vi "WF phase diversity_MATLAB_Correction_loop_AndorSDK_imq.vi"() -> ()   [LabVIEW 2018]
uses:
  <userlib>/WaveKit.lib/Controls/Wavefront Corrector states - ONE.ctl
  <userlib>/WaveKit.lib/Classes/WavefrontCorrector/WavefrontCorrector.lvclass
  <userlib>/WaveKit.lib/Classes/WavefrontCorrectorSet/WavefrontCorrectorSet.lvclass
  <vilib>/Analysis/1siggen.llb/Ramp Pattern by Samples.vi
  <vilib>/Utility/file.llb/Read From Spreadsheet File (DBL).vi
  <vilib>/Analysis/1siggen.llb/Ramp Pattern by Delta.vi
  <vilib>/Analysis/NI_AALBase.lvlib
panel:
  in  "Tab Control":T1(tab)
  in  "Offset command file":path=path "D:/SystemAlignment/system_aberration_20200627.dat"
  in  "Initial haso file":path=path "D:/SystemAlignment/system_aberration_residual_20200711.has"
  out "# of Phase":i32
  in  "DM configuration file":path=path "C:/Program Files (x86)/Imagine Optic/Configuration Files/WaveFrontCorrector_mirao52-e_0326.dat"
  out "DM Initial State":T2[](array[typedef])
  out "DM ActuatorsNumber":i32
  out "Error out":errorcluster
  in  "EMCCD trigger port":tag="Dev1/port0/line0"
  in  "COMMAND matrix path":path=path "D:/SystemAlignment/CM_20200711_0p5x6.aomc"
  out "Detector Y Pixels":i32
  out "Detector X Pixels":i32
  out "Return from Initialize":u32
  out "Return from SetTemperature":u32
  out "Calculated Exposure Value":sgl format="%.2f"
  out "Return from CheckTimings":u32
  in  "488 shutter":refnum<k7>(container)
  in  "?":bool
  in  "Initial Zer coeff":dbl[](array[numeric])=[0.2, 0.2]
  in  "Initial Zer index":dbl[](array[numeric])=[4.0, 5.0]
  out "Initial Zer coeff\nRandomly generated":dbl[](array[numeric])
  out "Initial Zer index (starting from 4)\nrandomly generated":dbl[](array[numeric])
  in  "aberration tolerance":dbl=0.1 format="%#_13g"
  in  "aberration threshold":dbl=0.25 format="%#_13g"
  in  "Initial Zern Coefficients":enum16{"input manually ", "randomly generated"}(ring)
  in  "max random order":i64=9
  in  "NOT YET: Data Acquisition Iteration #":i32=1
  in  "Index 5":i32[](array[numeric])=[3, 4, 5, 6, 7, 8]
  in  "Coef 4":sgl[](array[numeric])=[0.2, 0.0, 0.0, 0.0, 0.0, 0.0]
  in  "Index 4":i32[](array[numeric])=[3, 4, 5, 6, 7, 8]
  in  "Coef 3":sgl[](array[numeric])=[-0.2, -0.5, 0.0, 0.0, 0.0, 0.0]
  in  "Index 3":i32[](array[numeric])=[3, 4, 5, 6, 7, 8]
  in  "Coef 2":sgl[](array[numeric])=[0.2, 0.5, 0.0, 0.0, 0.0, 0.0]
  in  "Index 2":i32[](array[numeric])=[3, 4, 5, 6, 7, 8]
  in  "Zern coef in 5":sgl[](array[numeric])=[-0.2, 0.5, 0.0, 0.0, 0.0, 0.0]
  in  "base name":string="beads_test"
  in  "Imgs/phase":dbl=1.0
  in  "camera exposure time (s)":string="0.02"
  in  "# of Phase":i32=5
  in  "number of phase div image":dbl(ring)=2.0 items=["adding by step of 1 image"=1.0, "jump to 3 images"=0.9, "jump to 4 images"=2.0, "jump to 5 images"=2.9]
  in  "Metrics Type":T3(ring)=enum."norm DCT  - spectral domain 3: 0~r0"
  in  "Keep Reconstructed Defocus component?":bool
  in  "Run MATLAB or correction?":bool=TRUE
  in  "Number for average":u32=1
  in  "Zernike Order":u32=20
  in  "Iteration Number":u32=10
  in  "Gamma Value":dbl=1e-06
  in  "Crop Size of image":u32=512
  in  "Background Value":u32=290
  in  "Show Input":bool
  in  "Show Recon":bool=TRUE
  in  "Use GPU":bool=TRUE
  out "Cooling":i32
  in  "Trigger":u32(ring)=1 items=["Internal", "External"]
  in  "Cooler set to Temperature":i32=-60
  in  "Initialize EMCCD?":bool=TRUE
  in  "Turn off EMCCD when finished?":bool
  in  "Main Path":path=path "D:/Data"
  in  "Subfolder":string="Sample1"
  in  "Folder Name":string="Test"
  out "groundtruth image quality value":dbl
  out "aberrated image quality value":dbl
  out "Corrected Image Quality Value":dbl[](array[numeric])
  # "priority:\n1, flip, done by Min on 20200731? \n2, organize\n3, new matlab PD code\n4. isolate shutdown\n5. add \"galvo to andor\"\n6. setting log\n\n\n\n2 PhasDiv first\nif not, take 3 more or start over 5\n\n??: random iteration work??\n\nadd preview"
  # "If Pics/phase is 2:\npicture order:\n\noffset+aberr *2\nphase diversity *8\n\nground truth *1\noffset+aberr *1\ncorrected *2 but the last one cannot be seen in imagej"
  # "Andor Status"
  # "Random Input"
  # "Manual Input"
  # "Manual input sequence"
  # "Andor Camera Settings"
  # "Andor EMCCD Settings"
  # "MATLAB Settings"
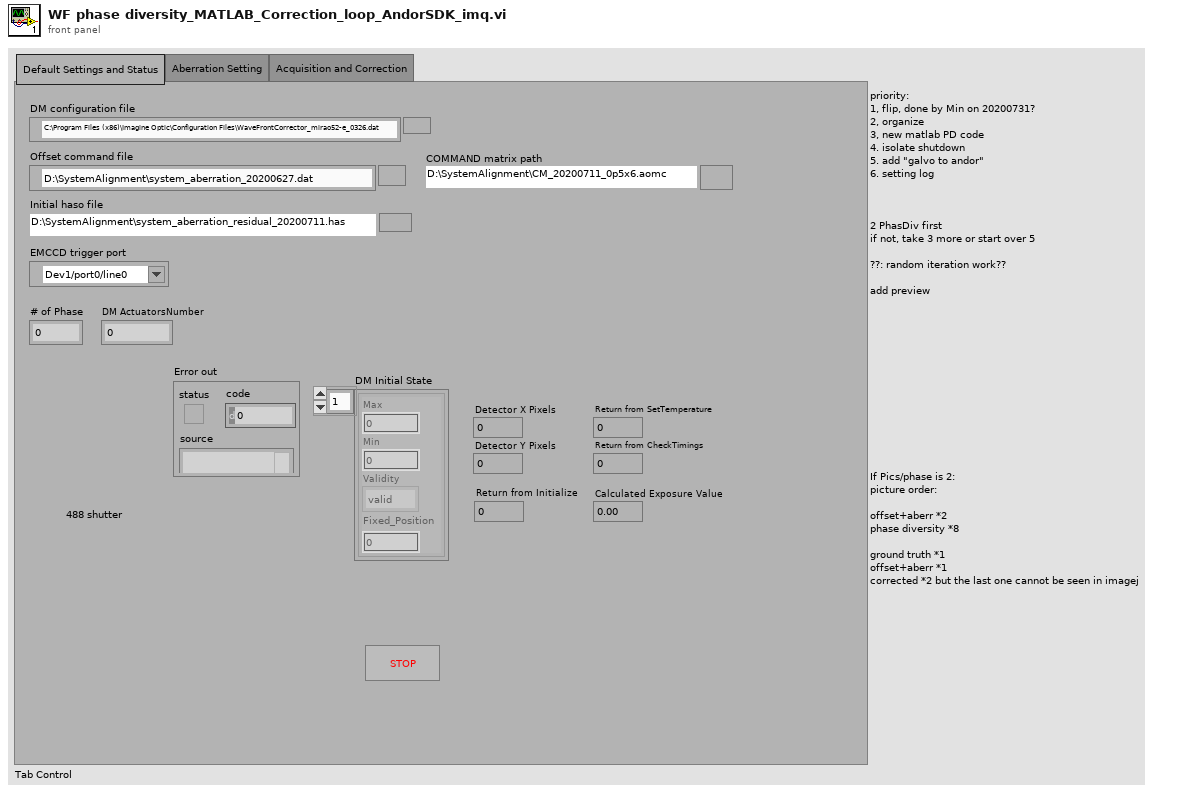
[diagram p1: front panel]
types:
  T1 = enum32{"Default Settings and Status", "Aberration Setting", "Acquisition and Correction"}
  T2 = typedef "Wavefront Corrector states - ONE.ctl" = cluster{"Max":sgl, "Min":sgl, "Validity":enum16{"valid", "fixed", "invalid"}, "Fixed_Position":sgl}
  T3 = enum16{" ", "max intensity", "mean intensity", "RMS contrast", "sharpness - image domain", "sharpness - spectral domain 1: 0~r0", "sharpness - spectral domain 2: 0.1*r0~0.5*r0", "norm DCT  - spectral domain 3: 0~r0"}
  T4 = typedef "Error Code Enum typedef.ctl" = enum32{"N/A (0)", "DRV_ERROR_CODES", "DRV_SUCCESS", "DRV_VXDNOTINSTALLED", "DRV_ERROR_SCAN", "DRV_ERROR_CHECK_SUM", "DRV_ERROR_FILELOAD", "DRV_UNKNOWN_FUNC", "DRV_ERROR_VXD_INIT", "DRV_ERROR_ADDRESS", "DRV_ERROR_PAGELOCK", "DRV_ERROR_PAGEUNLOCK", "DRV_ERROR_BOARDTEST", "DRV_ERROR_ACK", "DRV_ERROR_UP_FIFO", "DRV_ERROR_PATTERN", "N/A (16)", "DRV_ACQUISITION_ERRORS", "DRV_ACQ_BUFFER", "DRV_ACQ_DOWNFIFO_FULL", "DRV_PROC_UNKONWN_INSTRUCTION", "DRV_ILLEGAL_OP_CODE", "DRV_KINETIC_TIME_NOT_MET", "DRV_ACCUM_TIME_NOT_MET", "DRV_NO_NEW_DATA", "N/A (25)", "DRV_SPOOLERROR", "N/A (27)", "N/A (28)", "N/A (29)", "N/A (30)", "N/A (31)", "N/A (32)", "DRV_TEMPERATURE_CODES", "DRV_TEMPERATURE_OFF", "DRV_TEMPERATURE_NOT_STABILIZED", "DRV_TEMPERATURE_STABILIZED", "DRV_TEMPERATURE_NOT_REACHED", "DRV_TEMPERATURE_OUT_RANGE", "DRV_TEMPERATURE_NOT_SUPPORTED", "DRV_TEMPERATURE_DRIFT", "N/A (41)", "N/A (42)", "N/A (43)", "N/A (44)", "N/A (45)", "N/A (46)", "N/A (47)", "N/A (48)", "DRV_GENERAL_ERRORS", "DRV_INVALID_AUX", "DRV_COF_NOTLOADED", "DRV_FPGAPROG", "DRV_FLEXERROR", "DRV_GPIBERROR", "N/A (55)", "N/A (56)", "N/A (57)", "N/A (58)", "N/A (59)", "N/A (60)", "N/A (61)", "N/A (62)", "N/A (63)", "DRV_DATATYPE", "DRV_DRIVER_ERRORS", "DRV_P1INVALID", "DRV_P2INVALID", "DRV_P3INVALID", "DRV_P4INVALID", "DRV_INIERROR", "DRV_COFERROR", "DRV_ACQUIRING", "DRV_IDLE", "DRV_TEMPCYCLE", "DRV_NOT_INITIALIZED", "DRV_P5INVALID", "DRV_P6INVALID", "DRV_INVALID_MODE", "DRV_INVALID_FILTER", "DRV_I2CERRORS", "DRV_I2CDEVNOTFOUND", "DRV_I2CTIMEOUT", "DRV_P7INVALID", "N/A (84)", "N/A (85)", "N/A (86)", "N/A (87)", "N/A (88)", "N/A (89)", "DRV_IOCERROR", "DRV_VRMVERSIONERROR"}
  T5 = typedef "NI_Matrix.lvlib/RealMatrix.ctl" = dbl[][]
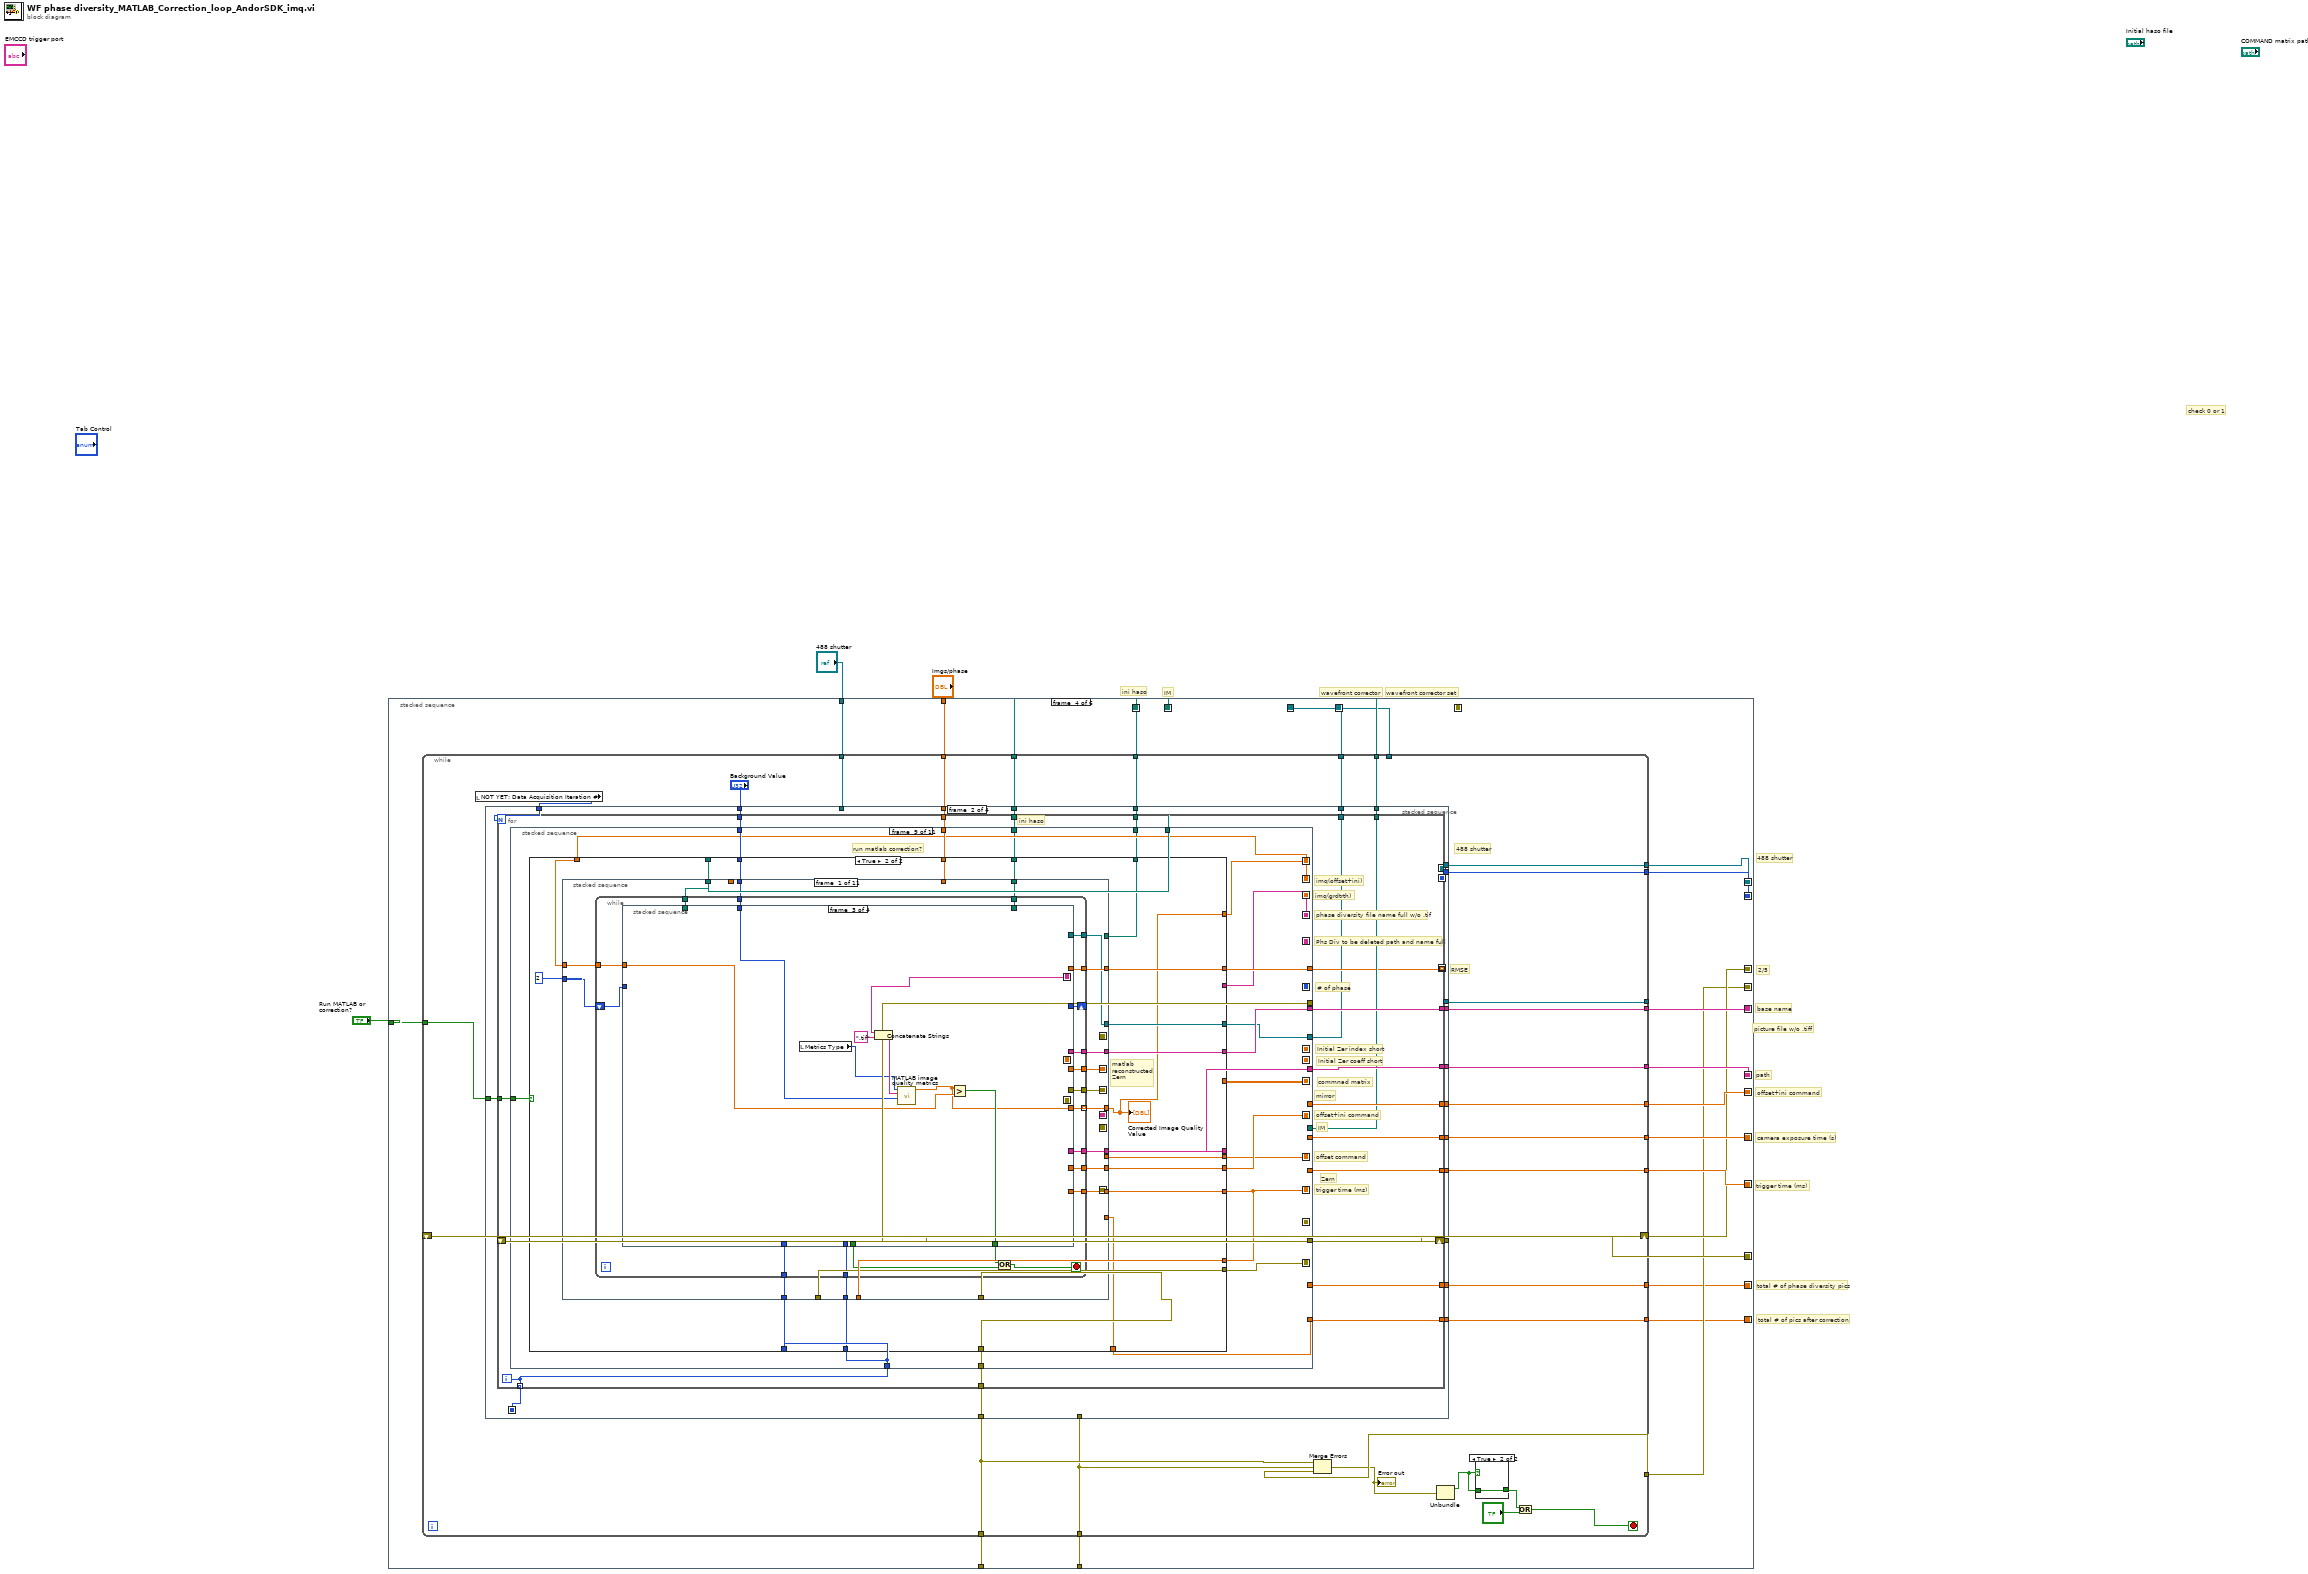
[diagram p0: block diagram]
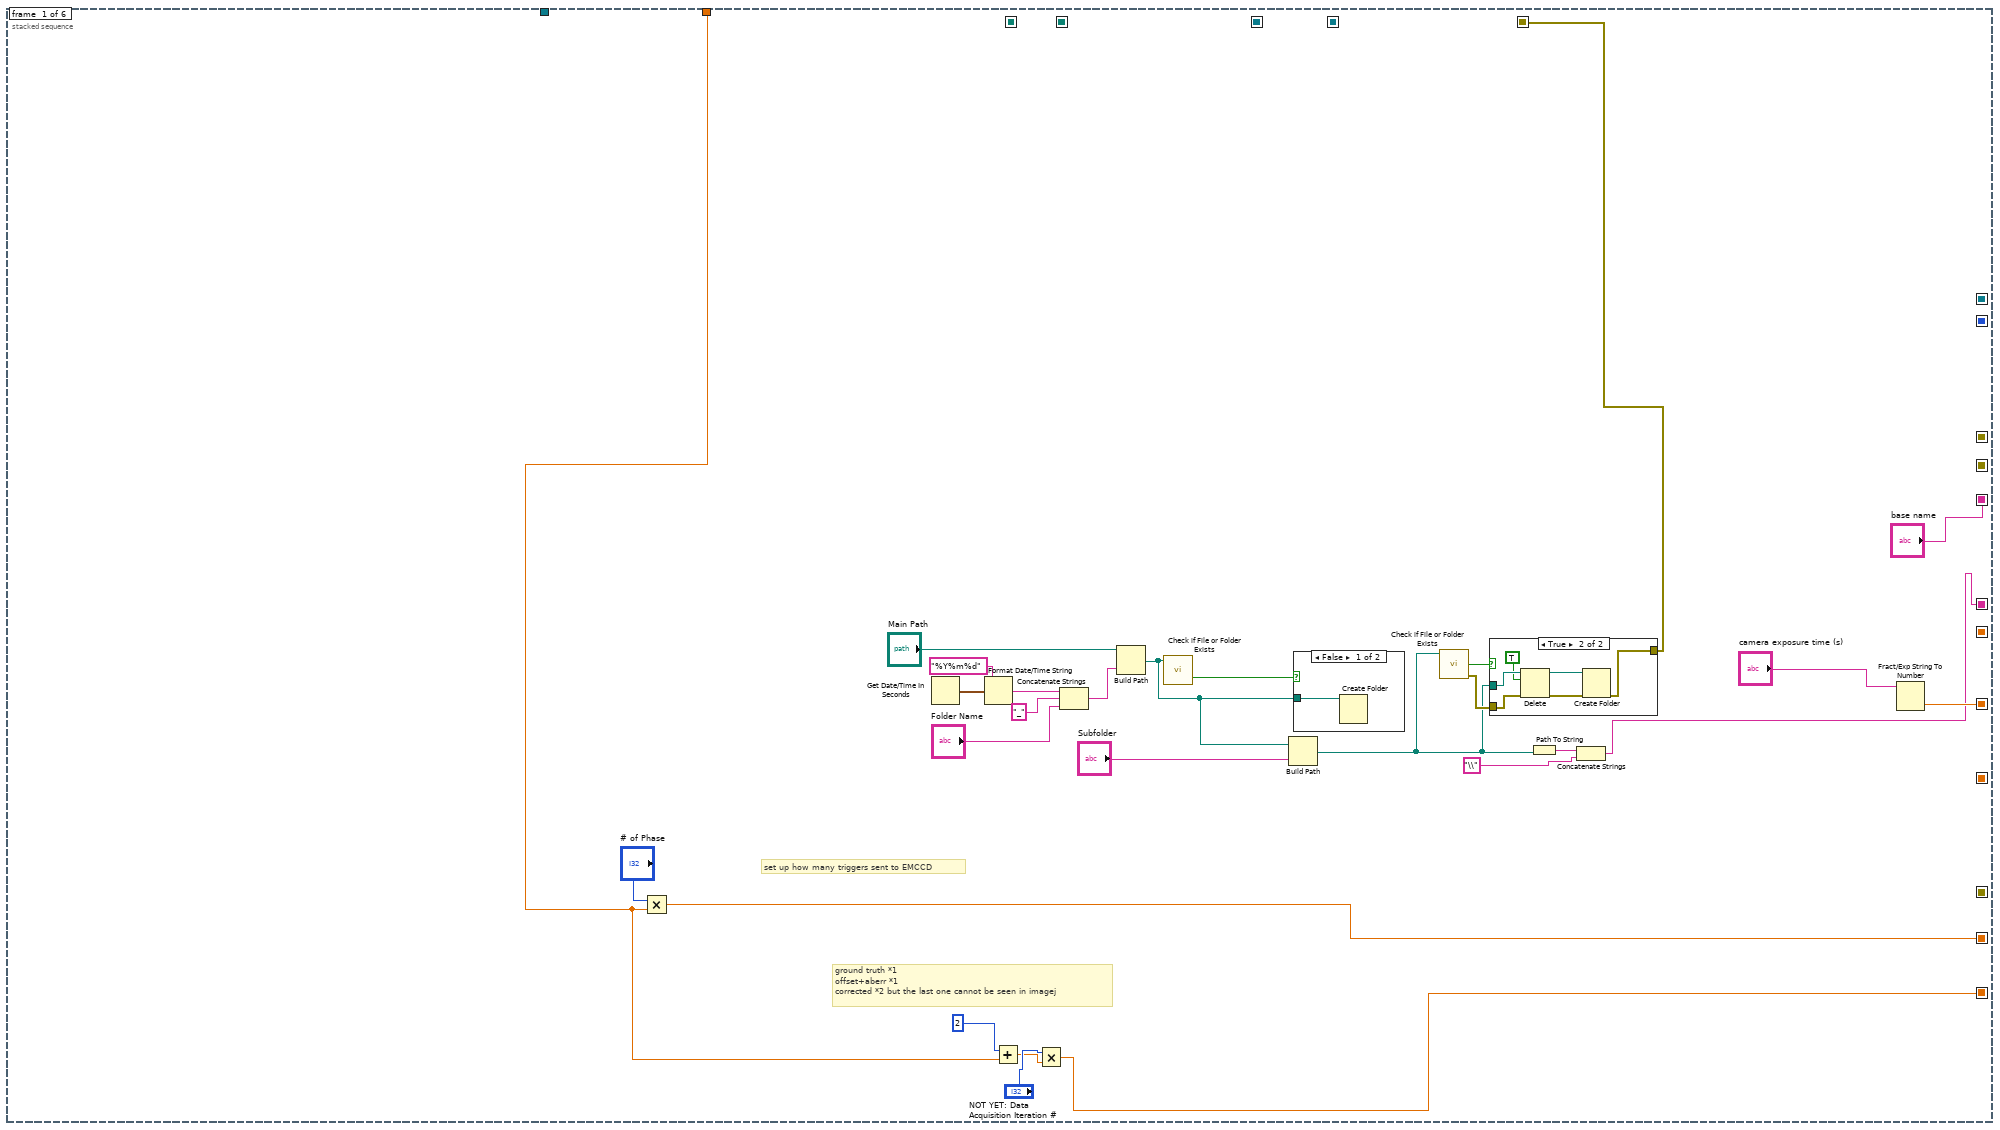
[diagram p2: hidden frame]
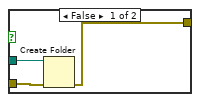
[diagram p3: hidden frame]
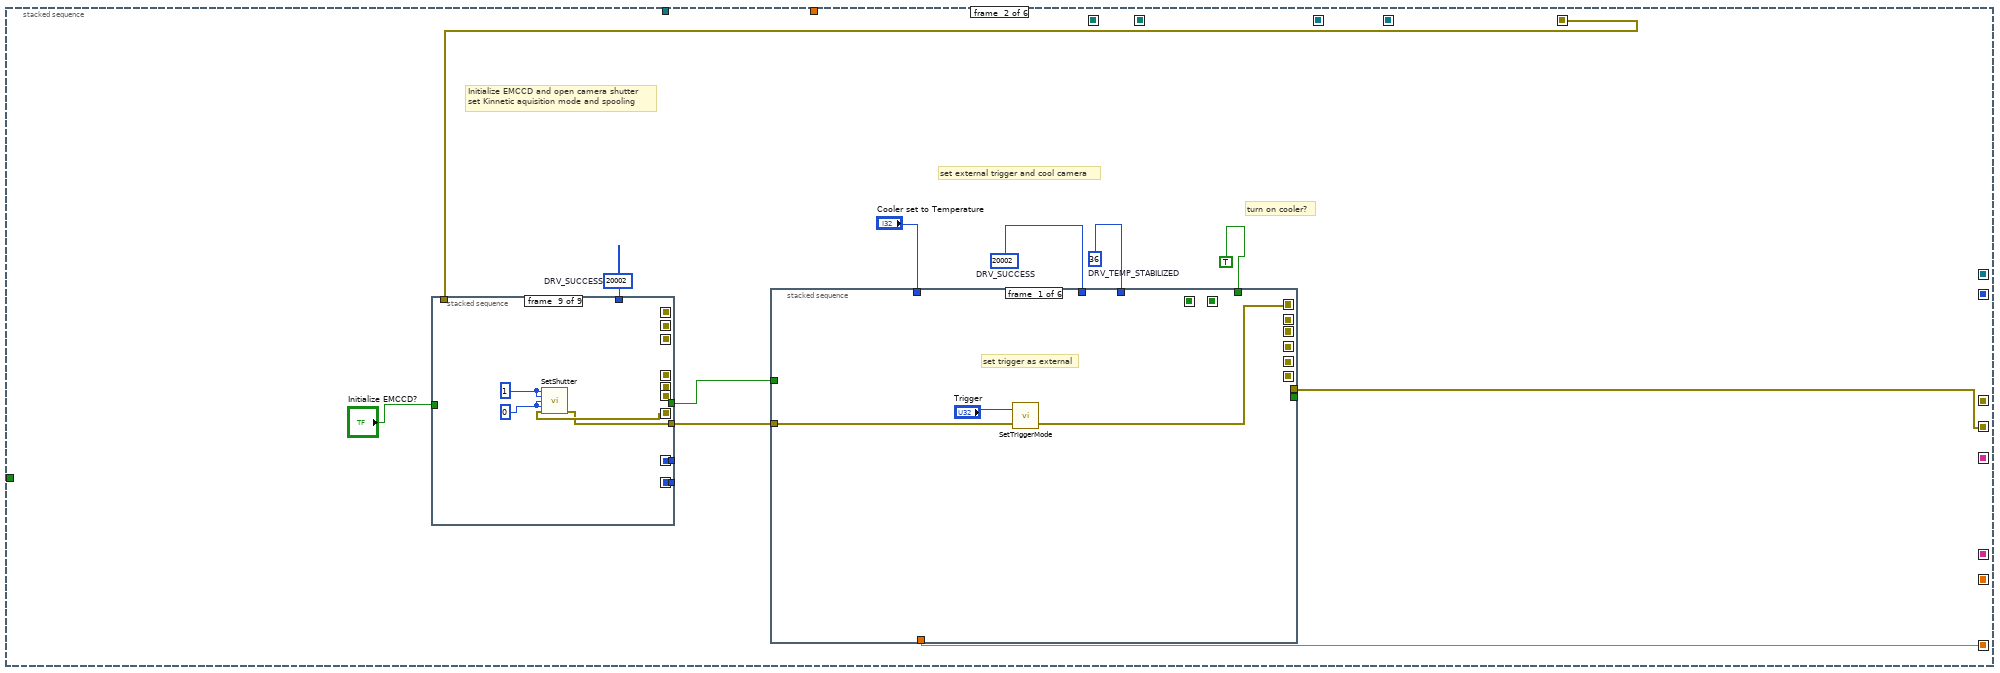
[diagram p5: hidden frame]
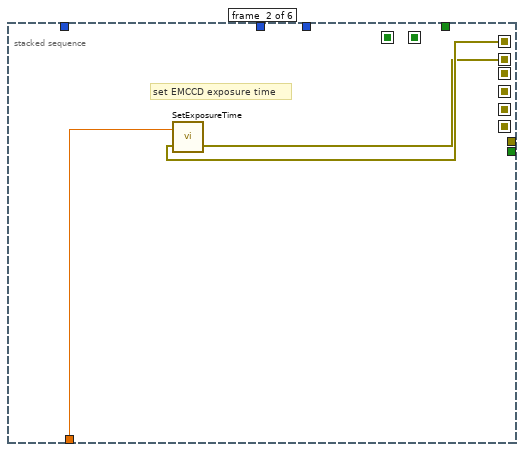
[diagram p6: hidden frame]
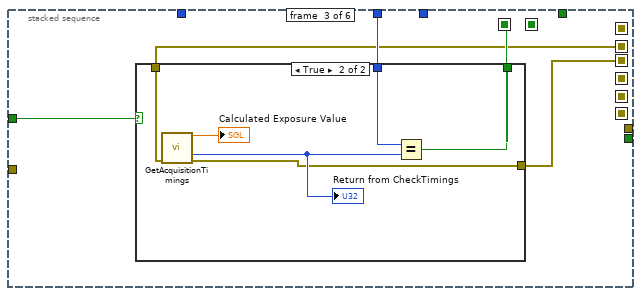
[diagram p7: hidden frame]
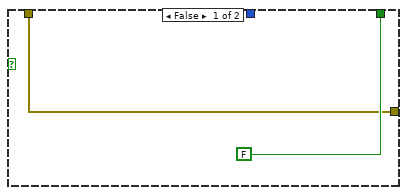
[diagram p8: hidden frame]
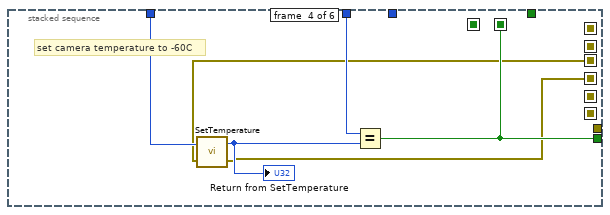
[diagram p9: hidden frame]
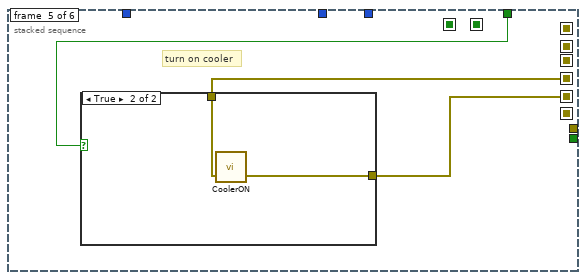
[diagram p10: hidden frame]
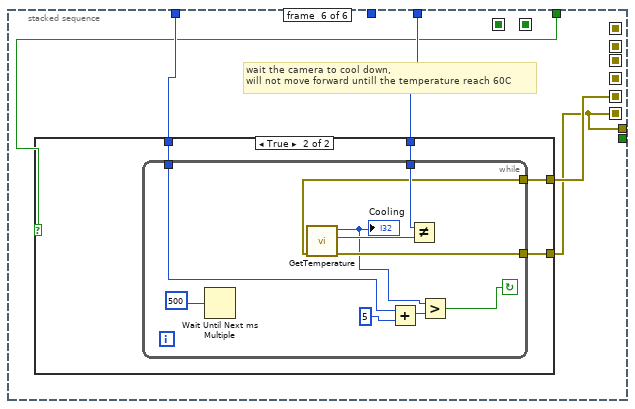
[diagram p12: hidden frame]
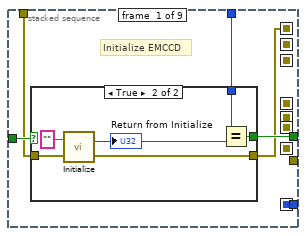
[diagram p14: hidden frame]
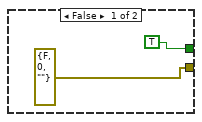
[diagram p15: hidden frame]
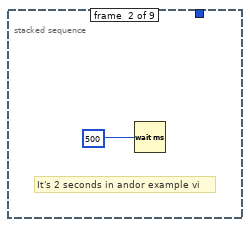
[diagram p16: hidden frame]
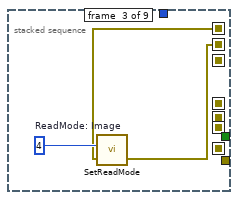
[diagram p17: hidden frame]
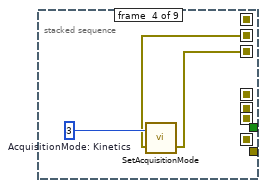
[diagram p18: hidden frame]
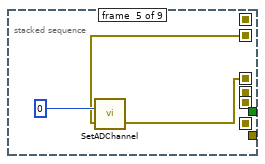
[diagram p19: hidden frame]
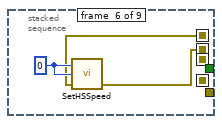
[diagram p20: hidden frame]
diagram:
  # "2/5"
  # "total # of phase diversity pics"
  # "picture file w/o .tiff"
  # "total # of pics after correction"
  # "wavefront corrector set"
  # "wavefront corrector"
  # "488 shutter"
  # "trigger time (ms)"
  # "offset+ini command"
  # "camera exposure time (s)"
  # "IM"
  # "ini haso"
  # "path"
  # "base name"
  # "check 0 or 1"
  n1 = stacked-sequence {
    seq-local: [w5 _ _ _ _ _] -> [_ _ _ w184 _ _]
    seq-local: ["base name" _ _ _ _ _] -> [_ _ _ w183 _ _]
    seq-local: [_ _ w164 _ _ _] -> [_ _ _ w165 _ _]
    seq-local: [_ _ w163 _ _ _] -> [_ _ _ w178 _ _]
    seq-local: [w27 _ _ _ _ _] -> [_ w44 _ w182 _ _]
    seq-local: [_ _ w149 _ _ _] -> [_ _ _ w170 _ _]
    seq-local: [_ _ _ w181 _ _] -> [_ _ _ _ _ _]
    seq-local: [_ _ _ w180 _ _] -> [_ _ _ _ _ _]
    seq-local: [_ _ _ w179 _ _] -> [_ _ _ _ _ w843]
    seq-local: [_ _ _ w173 _ _] -> [_ _ _ _ _ _]
    seq-local: [_ _ _ w176 _ _] -> [_ _ _ _ _ _]
    seq-local: [_ _ w148 _ _ _] -> [_ _ _ w171 _ w845]
    seq-local: [_ _ w147 _ _ _] -> [_ _ _ w169 _ w844]
    seq-local: [w24 _ _ _ _ _] -> [_ _ _ w166 _ _]
    seq-local: [_ w45 _ _ _ _] -> [_ _ w146 w168 _ _]
    seq-local: [w23 _ _ _ _ _] -> [_ _ _ w167 _ _]
    seq-local: [w4 _ _ _ _ _] -> [_ w41 _ _ _ _]
    tunnel: "Imgs/phase" -> [w21 _ _ w185 _ _]
    tunnel: "Run MATLAB or correction?" -> [_ _ _ w177 _ _]
    tunnel: [_ _ _ w175 _ _] -> _
    tunnel: [_ _ _ w174 _ _] -> _
    tunnel: "488 shutter" -> [_ _ _ w172 _ w846]
    frame #0 {
      # "set up how many triggers sent to EMCCD"
      # "ground truth *1\noffset+aberr *1\ncorrected *2 but the last one cannot be seen in imagej"
      n2 = Multiply(x="# of Phase", y=w21) -> (x*y=w23:dbl)
      n3 = Get Date/Time In Seconds() -> (seconds since 1Jan1904=w16:timestamp)
      n4 = Format Date/Time String(time format string (%c)="%Y%m%d", seconds (now)=w16) -> (date/time string=w17:string)  [unwired: 1 in]
      n5 = Add(x=2, y=w21) -> (x+y=w25:dbl)
      n6 = Multiply(x="NOT YET: Data Acquisition Iteration #", y=w25) -> (x*y=w24:dbl)
      n7 = Concatenate Strings(w17, "_", "Folder Name") -> (w18:string)
      n8 = Build Path(base path="Main Path", name or relative path=w18) -> (appended path=w20:path)
      n9 = call <vilib>:"Check if File or Folder Exists.vi"("path"=w20) -> ("file or folder exists?"=w14:bool)  [unwired: 8 in, 2 out]
      n10 = Build Path(base path=w20, name or relative path="Subfolder") -> (appended path=w6:path)
      n11 = case shown="False" w14 {
        tunnel: w20 -> [w40 _]
        frame False {
          n12 = Create Folder(path (use dialog)=w40) -> ()  [unwired: 2 in, 3 out]
        }
        frame True {
        }
      }
      n13 = call <vilib>:"Check if File or Folder Exists.vi"("path"=w6) -> ("error out"=w19:errorcluster, "file or folder exists?"=w15:bool)  [unwired: 8 in, 1 out]
      n14 = case shown="True" w15 {
        tunnel: w6 -> [w33 w38]
        tunnel: w19 -> [w32 w39]
        tunnel: [w31 w34] -> w4
        frame False {
          n15 = Create Folder(path (use dialog)=w33, error in=w32) -> (error out=w31:errorcluster)  [unwired: 1 in, 2 out]
        }
        frame True {
          n16 = Delete(path (use dialog)=w38, entire hierarchy (F)=TRUE, error in=w39) -> (deleted path=w36:path, error out=w35:errorcluster)  [unwired: 2 in, 1 out]
          n17 = Create Folder(path (use dialog)=w36, error in=w35) -> (error out=w34:errorcluster)  [unwired: 1 in, 2 out]
        }
      }
      n18 = Path To String(path=w6) -> (string=w8:string)
      n19 = Concatenate Strings(w8, "\\") -> (w5:string)
      n20 = Fract/Exp String To Number(string="camera exposure time (s)") -> (number=w27:dbl)  [unwired: 3 in, 1 out]
    }
    frame #1 {
      w47 = 36  # DRV_TEMP_STABILIZED
      w49 = 20002  # DRV_SUCCESS
      w51 = 20002  # DRV_SUCCESS
      # "turn on cooler?"
      # "set external trigger and cool camera"
      # "Initialize EMCCD and open camera shutter\nset Kinnetic aquisition mode and spooling"
      n21 = stacked-sequence {
        seq-local: [_ _ _ _ _ _ _ w135 _] -> [_ _ _ _ _ _ _ _ _]
        seq-local: [_ _ _ _ _ _ _ w137 _] -> [_ _ _ _ _ _ _ _ _]
        seq-local: [w105 _ _ _ _ _ _ _ _] -> [_ _ w118 _ _ _ _ _ _]
        seq-local: [_ _ w117 _ _ _ _ _ _] -> [_ _ _ w121 _ _ _ _ _]
        seq-local: [_ _ _ w120 _ _ _ _ _] -> [_ _ _ _ w123 _ _ _ _]
        seq-local: [_ _ _ _ w124 _ _ _ _] -> [_ _ _ _ _ w127 _ _ _]
        seq-local: [_ _ _ _ _ w126 _ _ _] -> [_ _ _ _ _ _ w131 _ _]
        seq-local: [_ _ _ _ _ _ w129 _ _] -> [_ _ _ _ _ _ _ w140 _]
        seq-local: [_ _ _ _ _ _ _ w138 _] -> [_ _ _ _ _ _ _ _ w143]
        tunnel: w51 -> [w107 _ _ _ _ _ _ _ _]
        tunnel: [w106 _ _ _ _ _ _ _ _] -> w50
        tunnel: [_ _ _ _ _ _ _ w135 _] -> _
        tunnel: [_ _ _ _ _ _ _ w137 _] -> _
        tunnel: [_ _ _ _ _ _ _ _ w142] -> w46
        tunnel: "Initialize EMCCD?" -> [w104 _ _ _ _ _ _ _ _]
        tunnel: w41 -> [w103 _ _ _ _ _ _ _ _]
        frame #0 {
          # "Initialize EMCCD"
          n22 = case shown="True" w104 {
            tunnel: w107 -> [_ w113]
            tunnel: [TRUE w112] -> w106
            tunnel: [errorcluster {"status"=FALSE, "code"=0, "source"=""} ("Error in 2") w111] -> w105
            tunnel: w103 -> [_ w110]
            frame False {
            }
            frame True {
              n23 = call <userlib>:"Initialize.vi"("error in (no error)"=w110, "directory (\"\")"="" ("directory (\"\")")) -> ("error out"=w111:errorcluster, "DLL error code"=w115:u32)
              "Return from Initialize" <- w115
              n24 = Equal?(x=w113, y=w115) -> (x = y?=w112:bool)
            }
          }
        }
        frame #1 {
          # "It's 2 seconds in andor example vi"
          n25 = Wait (ms)(milliseconds to wait=u32 500) -> ()  [unwired: 1 out]
        }
        frame #2 {
          w119 = u16 4  # ReadMode: Image
          n26 = call <userlib>:"SetReadMode.vi"("error in (no error)"=w118, "mode"=w119) -> ("error out"=w117:errorcluster)  [unwired: 1 out]
        }
        frame #3 {
          w122 = u16 3  # AcquisitionMode: Kinetics
          n27 = call <userlib>:"SetAcquisitionMode.vi"("error in (no error)"=w121, "mode"=w122) -> ("error out"=w120:errorcluster)  [unwired: 1 out]
        }
        frame #4 {
          n28 = call <userlib>:"SetADChannel.vi"("error in (no error)"=w123, "channel"=0) -> ("error out"=w124:errorcluster)  [unwired: 1 out]
        }
        frame #5 {
          w128 = 0
          n29 = call <userlib>:"SetHSSpeed.vi"("error in (no error)"=w127, "index"=w128, "type"=w128) -> ("error out"=w126:errorcluster)  [unwired: 1 in, 1 out]
        }
        frame #6 {
          n30 = call <userlib>:"GetNumberVSSpeeds.vi"("error in (no error)"=w131) -> ("error out"=w130:errorcluster, "number"=w134:i32)  [unwired: 2 in, 1 out]
          n31 = Subtract(x=w134, y=1) -> (x-y=w132:i32)
          n32 = call <userlib>:"SetVSSpeed.vi"("error in (no error)"=w130, "index"=w132) -> ("error out"=w129:errorcluster)  [unwired: 1 out]
        }
        frame #7 {
          w141 = 1
          n33 = call <userlib>:"GetDetector.vi"("error in (no error)"=w140) -> ("error out"=w139:errorcluster, "ypixels"=w136:i32, "xpixels"=w137:i32)  [unwired: 3 in, 1 out]
          "Detector Y Pixels" <- w136
          "Detector X Pixels" <- w137
          n34 = Max & Min(x=w137, y=w136) -> (min(x,y)=w135:i32)  [unwired: 1 out]
          n35 = call <userlib>:"SetImage.vi"("hbin"=w141, "vbin"=w141, "hstart"=w141, "hend"=w135, "vstart"=w141, "vend"=w135, "error in (no error)"=w139) -> ("error out"=w138:errorcluster)  [unwired: 19 in, 1 out]
        }
        frame #8 {
          w144 = 0
          w145 = 1
          n36 = call <userlib>:"SetShutter.vi"("type"=w145, "mode"=w145, "closingtime"=w144, "openingtime"=w144, "error in (no error)"=w143) -> ("error out"=w142:errorcluster)  [unwired: 9 in, 1 out]
        }
      }
      n37 = stacked-sequence {
        seq-local: [_ _ w60 _ _ _] -> [_ _ _ _ _ _]
        seq-local: [_ _ _ w73 _ _] -> [_ _ _ _ _ _]
        seq-local: [w52 _ _ _ _ _] -> [_ w57 _ _ _ _]
        seq-local: [_ w56 _ _ _ _] -> [_ _ w59 _ _ _]
        seq-local: [_ _ w58 _ _ _] -> [_ _ _ w72 _ _]
        seq-local: [_ _ _ w71 _ _] -> [_ _ _ _ w79 _]
        seq-local: [_ _ _ _ w78 _] -> [_ _ _ _ _ w85]
        seq-local: [_ _ _ _ _ w83] -> [_ _ _ _ _ _]
        tunnel: w49 -> [_ _ w62 w76 _ _]
        tunnel: "Cooler set to Temperature" -> [_ _ _ w74 _ w86]
        tunnel: w47 -> [_ _ _ _ _ w87]
        tunnel: [_ _ _ w73 _ _] -> _
        tunnel: w50 -> [_ _ w61 _ _ _]
        tunnel: w46 -> [w53 _ _ _ _ _]
        tunnel: [_ _ _ _ _ w83] -> w45
        tunnel: w44 -> [_ w55 _ _ _ _]
        tunnel: TRUE -> [_ _ _ _ w77 w84]
        frame #0 {
          # "set trigger as external"
          n38 = call <userlib>:"SetTriggerMode.vi"("error in (no error)"=w53, "mode"="Trigger") -> ("error out"=w52:errorcluster)  [unwired: 1 out]
        }
        frame #1 {
          # "set EMCCD exposure time"
          n39 = call <userlib>:"SetExposureTime.vi"("error in (no error)"=w57, "time"=w55) -> ("error out"=w56:errorcluster)  [unwired: 1 out]
        }
        frame #2 {
          n40 = case shown="True" w61 {
            tunnel: w62 -> [_ w68]
            tunnel: [FALSE w70] -> w60
            tunnel: w59 -> [w63 w66]
            tunnel: [w63 w65] -> w58
            frame False {
            }
            frame True {
              n41 = call <userlib>:"GetAcquisitionTimings.vi"("error in (no error)"=w66) -> ("exposure"=→"Calculated Exposure Value":sgl, "DLL error code"=w67:u32, "error out"=w65:errorcluster)  [unwired: 10 in, 2 out]
              "Return from CheckTimings" <- w67
              n42 = Equal?(x=w68, y=w67) -> (x = y?=w70:bool)
            }
          }
        }
        frame #3 {
          # "set camera temperature to -60C"
          n43 = call <userlib>:"SetTemperature.vi"("error in (no error)"=w72, "temperature"=w74) -> ("error out"=w71:errorcluster, "DLL error code"=w75:u32)
          "Return from SetTemperature" <- w75
          n44 = Equal?(x=w76, y=w75) -> (x = y?=w73:bool)
        }
        frame #4 {
          # "turn on cooler"
          n45 = case shown="True" w77 {
            tunnel: w79 -> [w80 w82]
            tunnel: [w80 w81] -> w78
            frame False {
            }
            frame True {
              n46 = call <userlib>:"CoolerON.vi"("error in (no error)"=w82) -> ("error out"=w81:errorcluster)  [unwired: 1 in, 1 out]
            }
          }
        }
        frame #5 {
          # "wait the camera to cool down,\nwill not move forward untill the temperature reach 60C"
          n47 = case shown="True" w84 {
            tunnel: w87 -> [_ w92]
            tunnel: w86 -> [_ w91]
            tunnel: w85 -> [w88 w90]
            tunnel: [w88 w89] -> w83
            frame False {
            }
            frame True {
              n48 = while {
                tunnel: w92 -> [w101]
                tunnel: w91 -> [w96]
                tunnel: w90 -> [w99]
                tunnel: [w98] -> w89
                stop <- w93 continue-if-true
                n49 = Wait Until Next ms Multiple(millisecond multiple=u32 500) -> ()  [unwired: 1 out]
                n50 = call <userlib>:"GetTemperature.vi"("error in (no error)"=w99) -> ("error out"=w98:errorcluster, "status"=w100:T4, "temperature"=w94:i32)  [unwired: 3 in, 1 out]
                "Cooling" <- w94
                n51 = Add(x=w96, y=5) -> (x+y=w95:i32)
                n52 = Not Equal?(x=w101, y=w100) -> ()  [unwired: 1 out]
                n53 = Greater?(x=w94, y=w95) -> (0:w93:bool)
              }
            }
          }
        }
      }
    }
    frame #2 {
      # "Initialize CASAO"
      n54 = call <userlib>:"LVClass_WavefrontCorrectorSet ctor.vi"("WavefrontCorrectorSet in"=refnum<class "WavefrontCorrectorSet.lvclass"> refnum, "PathToWavefrontCorrectorSetupFile"="DM configuration file", "error in (no error)"=w146) -> ("WavefrontCorrectorSet out"=w153:refnum<class "WavefrontCorrectorSet.lvclass">, "error out"=w162:errorcluster)  [unwired: 11 in]
      n55 = call <userlib>:"LVClass_WavefrontCorrector ctor.vi"("WavefrontCorrector in"=refnum<class "WavefrontCorrector.lvclass"> refnum, "PathToWavefrontCorrectorSetupFile"="DM configuration file", "error in (no error)"=w162) -> ("WavefrontCorrector out"=w157:refnum<class "WavefrontCorrector.lvclass">, "error out"=w156:errorcluster)  [unwired: 11 in]
      n56 = call <userlib>:"LVClass_WavefrontCorrector Init.vi"("WavefrontCorrector in"=w157, "set_init_state_from_config_file"=TRUE, "error in (no error)"=w156) -> ("WavefrontCorrector out"=w151:refnum<class "WavefrontCorrector.lvclass">, "error out"=w155:errorcluster)  [unwired: 11 in]
      n57 = call <userlib>:"LVClass_WavefrontCorrectorSet get nb of actuators.vi"("WavefrontCorrectorSet in"=w153, "error in (no error)"=w155) -> ("WavefrontCorrectorSet out"=w147:refnum<class "WavefrontCorrectorSet.lvclass">, "ActuatorsNumber"=→"DM ActuatorsNumber":i32, "error out"=w152:errorcluster)  [unwired: 11 in]
      n58 = call <userlib>:"LVClass_WavefrontCorrector Get Current Preferences.vi"("WavefrontCorrector in"=w151, "error in (no error)"=w152) -> ("WavefrontCorrector out"=w148:refnum<class "WavefrontCorrector.lvclass">, "Mirror preferences.Wavefront Corrector State"=→"DM Initial State":T2[], "error out"=w149:errorcluster)  [unwired: 10 in, 1 out]
      n59 = local read "COMMAND matrix path"() -> (w163:path)
      n60 = local read "Initial haso file"() -> (w164:path)
    }
    frame #3 {
      n61 = while {
        tunnel: w185 -> [w214]
        tunnel: w184 -> [w213]
        tunnel: w183 -> [w212]
        tunnel: w165 -> [w211]
        tunnel: w182 -> [w210]
        tunnel: [w208] -> w181
        tunnel: [w207] -> w180
        tunnel: w178 -> [w205]
        tunnel: w177 -> [w204]
        tunnel: [w203] -> w176
        tunnel: [w202] -> _
        tunnel: [w200] -> w175
        tunnel: [w201] -> w174
        shift-right: [w206] -> w179
        shift-left: w170 -> [w209]
        tunnel: [w199] -> w173
        tunnel: w172 -> [w198]
        tunnel: w171 -> [w197]
        tunnel: w169 -> [_]
        tunnel: w168 -> [w195]
        tunnel: w167 -> [w189]
        tunnel: w166 -> [w188]
        tunnel: w165 -> [w186]
        stop <- w191 stop-if-true
        # "488 shutter"
        # "RMSE"
        n62 = local read "NOT YET: Data Acquisition Iteration #"() -> (w196:i32)
        n63 = stacked-sequence {
          seq-local: [_ w232 _ _] -> [_ _ _ w835]
          seq-local: [_ w231 _ _] -> [_ _ _ _]
          seq-local: [w219 _ _ _] -> [_ _ w831 _]
          seq-local: [w220 _ _ _] -> [_ _ w830 _]
          tunnel: w214 -> [_ w244 _ _]
          tunnel: w213 -> [_ w243 _ w834]
          tunnel: w212 -> [_ w242 _ w833]
          tunnel: w211 -> [_ w241 _ _]
          tunnel: w210 -> [_ w240 _ _]
          tunnel: w209 -> [_ w239 _ _]
          tunnel: [_ w238 _ _] -> w208
          tunnel: [_ w237 _ _] -> w207
          tunnel: [_ w236 _ _] -> w206
          tunnel: w205 -> [_ w235 _ _]
          tunnel: w204 -> [_ w234 _ _]
          tunnel: w196 -> [_ w233 _ _]
          tunnel: [_ _ w829 _] -> w202
          tunnel: [_ _ w828 _] -> w203
          tunnel: [_ _ _ w832] -> w200
          tunnel: [_ w230 _ _] -> w201
          tunnel: [w219 _ _ _] -> w199
          tunnel: w198 -> [w218 _ _ _]
          tunnel: w197 -> [_ w229 _ _]
          tunnel: w189 -> [_ w228 _ _]
          tunnel: w188 -> [_ w227 _ _]
          tunnel: "Background Value" -> [_ w226 _ _]
          tunnel: w186 -> [_ w225 _ _]
          frame #0 {
            # "open the shutter of 488nm laser"
            n64 = property class="MG17Motor"(reference=w218, "HWSerialNum"=85819115.0) -> (reference out=w224:refnum<k7>)  [unwired: 1 in, 1 out]
            n65 = invoke class="MG17Motor" method="StartCtrl"(reference=w224) -> (reference out=w222:refnum<k7>)  [unwired: 2 in, 2 out]
            n66 = invoke class="MG17Motor" method="SC_Enable"(reference=w222, "lChanID"=0) -> (reference out=w219:refnum<k7>, "lChanID"=w220:i32)  [unwired: 2 in, 2 out]
          }
          frame #1 {
            n67 = for {
              N: w233 -> [_]
              tunnel: w244 -> [w263]
              tunnel: w243 -> [w262]
              tunnel: w242 -> [w261]
              tunnel: w241 -> [w260]
              tunnel: w240 -> [w259]
              tunnel: [w257] -> w238
              tunnel: [w256] -> w237
              tunnel: w235 -> [w254]
              tunnel: w234 -> [w253]
              shift-right: [w255] -> w236
              shift-left: w239 -> [w258]
              tunnel: [w252] -> w232 mode=indexing
              tunnel: [w251] -> w231 mode=indexing
              tunnel: [w250] -> w230
              tunnel: w229 -> [w249]
              tunnel: w228 -> [w248]
              tunnel: w227 -> [w247]
              tunnel: w226 -> [w246]
              tunnel: w225 -> [w245]
              i -> [w251]
              # "imq(grdtrth)"
              # "imq(offset+ini)"
              # "Phs Div to be deleted path and name full"
              # "phase diversity file name full w/o .tif"
              # "# of phase"
              # "trigger time (ms)"
              # "offset+ini command"
              # "Initial Zer coeff short"
              # "Initial Zer index short"
              # "mirror"
              # "Zern"
              # "commnad matrix"
              # "ini haso"
              # "IM"
              # "offset command"
              n68 = stacked-sequence {
                seq-local: [_ w275 _ _ _ _ _ _ _ _ _] -> [_ _ w295 _ w423 _ _ w482 w536 _ _]
                seq-local: [_ _ w293 _ _ _ _ _ _ _ _] -> [_ _ _ _ w422 _ _ _ w538 _ _]
                seq-local: [_ _ w291 _ _ _ _ _ _ _ _] -> [_ _ _ _ w421 _ _ _ _ _ _]
                seq-local: [_ _ w284 _ _ _ _ _ _ _ _] -> [_ _ _ _ w418 _ _ _ _ _ _]
                seq-local: [w266 _ _ _ _ _ _ _ _ _ _] -> [_ _ w281 _ _ _ _ _ _ _ _]
                seq-local: [w265 _ _ _ _ _ _ _ _ _ _] -> [_ _ w280 _ _ _ _ _ _ _ _]
                seq-local: [_ _ w279 _ _ _ _ _ _ _ _] -> [_ _ _ _ _ _ _ w484 w542 _ _]
                seq-local: [_ _ _ _ w417 _ _ _ _ _ _] -> [_ _ _ _ _ w467 _ w487 w529 _ _]
                seq-local: [_ _ _ _ w416 _ _ _ _ _ _] -> [_ _ _ _ _ _ _ _ w540 _ _]
                seq-local: [_ _ _ _ _ _ w471 _ _ _ _] -> [_ _ _ _ _ _ _ _ w532 _ _]
                seq-local: [_ _ _ w410 _ _ _ _ _ _ _] -> [_ _ _ _ _ _ _ _ _ w773 _]
                seq-local: [_ _ _ _ _ _ _ w483 _ _ _] -> [_ _ _ _ _ _ _ _ _ _ w808]
                seq-local: [_ _ _ _ _ _ _ w481 _ _ _] -> [_ _ _ _ _ _ _ _ w530 _ w804]
                seq-local: [_ _ _ _ _ _ _ _ w525 _ _] -> [_ _ _ _ _ _ _ _ _ _ w800]
                tunnel: w263 -> [_ _ w288 _ w426 _ _ _ w541 _ _]
                tunnel: w262 -> [_ _ w289 w413 w425 _ w478 w490 w544 _ w792]
                tunnel: w261 -> [_ _ w290 w412 w424 _ w480 w489 w545 _ w791]
                tunnel: w260 -> [_ _ w287 _ _ _ _ _ w527 _ _]
                tunnel: w254 -> [_ _ w286 _ w420 _ _ _ _ _ _]
                tunnel: w259 -> [_ _ _ _ w419 _ _ _ _ _ _]
                tunnel: w258 -> [_ _ w285 _ _ _ _ _ _ _ _]
                tunnel: [_ _ _ _ w416 _ _ _ _ _ _] -> w255
                tunnel: [_ _ w279 _ _ _ _ _ _ _ _] -> w257
                tunnel: [_ _ _ _ w417 _ _ _ _ _ _] -> w256
                tunnel: w254 -> [_ _ _ _ _ _ _ _ w543 _ _]
                tunnel: w253 -> [_ _ _ _ _ _ _ _ w539 _ _]
                tunnel: w251 -> [_ _ w278 w409 _ _ w479 w488 w528 _ _]
                tunnel: [_ _ _ _ _ _ _ _ w537 _ _] -> w252
                tunnel: [_ _ _ _ _ _ _ _ w535 _ _] -> w250
                tunnel: w249 -> [_ _ _ _ w415 _ _ w486 w534 _ _]
                tunnel: w248 -> [_ _ _ w414 _ _ _ _ _ w771 _]
                tunnel: w247 -> [_ _ _ _ _ _ _ _ w533 _ _]
                tunnel: w246 -> [_ _ _ _ _ _ _ w485 w531 _ _]
                tunnel: w245 -> [_ _ _ _ _ _ _ _ w526 _ _]
                frame #0 {
                  # "generate initial aberration (aberr to correct)"
                  n69 = case shown="\"randomly generated\"" "Initial Zern Coefficients" {
                    tunnel: ["Initial Zer index" w272] -> w266
                    tunnel: ["Initial Zer coeff" w271] -> w265
                    tunnel: "max random order" -> [_ w270]
                    frame "input manually " {
                    }
                    frame "randomly generated" {
                      # "generate random zernike index and coefficient arrays"
                      n70 = call "Random Aberration Array Generator.vi"("max random order"=w270, "aberration tolerance"="aberration tolerance", "aberration threshold"="aberration threshold") -> ("Zer coeff"=w271:dbl[], "Zer index (starting from 3)"=w272:dbl[])  [unwired: 7 in]
                      "Initial Zer index (starting from 4)\nrandomly generated" <- w272
                      "Initial Zer coeff\nRandomly generated" <- w271
                    }
                  }
                }
                frame #1 {
                  # "read in offset command"
                  n71 = call-poly <vilib>:"Read From Spreadsheet File.vi"("format (%.3f)"="%.8f", "file path (dialog if empty)"="Offset command file") -> ("first row"=w275:dbl[])  [unwired: 5 in, 4 out]
                }
                frame #2 {
                  w300 = 0.0
                  # "ini zern coeff"
                  # "offset+ini command"
                  # "Zern coeff"
                  # "Zern index"
                  # "calculate the command:\nfor phase diversity"
                  n72 = Array Size(array="Index 2") -> (size(s)=w298:i32)
                  n73 = call-poly <vilib>:"Ramp Pattern.vi"("start"=w300, "end"=w300, "samples"=w298) -> ("Ramp Pattern"=w297:dbl[])  [unwired: 7 in, 1 out]
                  n74 = Build Array(w297, "Index 2", "Index 3", "Index 4", "Index 5") -> (w282:T5)
                  n75 = Build Array(w297, "Coef 2", "Coef 3", "Coef 4", "Zern coef in 5") -> (w301:T5)
                  n76 = Transpose Matrix(1:w301) -> (0:w294:T5)
                  n77 = Transpose Matrix(1:w282) -> (0:w292:T5)
                  n78 = Array Size(array=w282) -> (size(s)=w283:i32[])
                  n79 = Index Array(array=w283, index=1) -> (element=w291:i32)
                  "# of Phase" <- w291
                  n80 = stacked-sequence {
                    seq-local: [w310 _ _] -> [_ w328 w394]
                    seq-local: [w311 _ _] -> [_ w322 _]
                    seq-local: [_ w321 _] -> [_ _ w391]
                    seq-local: [w309 _ _] -> [_ w320 _]
                    tunnel: w291 -> [_ w333 _]
                    tunnel: w281 -> [w318 _ _]
                    tunnel: w280 -> [w317 w323 _]
                    tunnel: w286 -> [w316 w330 _]
                    tunnel: w295 -> [w314 _ _]
                    tunnel: w292 -> [_ w332 _]
                    tunnel: w294 -> [_ w331 _]
                    tunnel: w287 -> [w313 w329 _]
                    tunnel: [_ w327 _] -> w293
                    tunnel: w290 -> [_ w325 w392]
                    tunnel: w289 -> [_ w326 w393]
                    tunnel: w288 -> [_ w324 _]
                    tunnel: w285 -> [w312 _ _]
                    tunnel: [_ _ w390] -> w284
                    tunnel: [w310 _ _] -> w279
                    tunnel: w278 -> [_ w319 w388]
                    frame #0 {
                      n81 = call "zern2command_test.vi"("Initial haso file"=w313, "error in (no error)"=w312, "interaction matrix file"=w316, "Zern coef in"=w317, "Zern index in"=w318) -> ("error out"=w311:errorcluster, "Zern coef out"=w309:sgl[], "Offset positions"=w315:sgl[])  [unwired: 4 in]
                      n82 = Add(x=w315, y=w314) -> (x+y=w310:dbl[])
                    }
                    frame #1 {
                      n83 = for {
                        N: w333 -> [w336]
                        tunnel: w332 -> [w349] mode=indexing
                        tunnel: w331 -> [w348] mode=indexing
                        tunnel: w330 -> [w347]
                        tunnel: w329 -> [w346]
                        tunnel: w328 -> [w345]
                        tunnel: [w344] -> w327 mode=indexing
                        tunnel: w326 -> [w343]
                        tunnel: w325 -> [w342]
                        tunnel: w324 -> [w341]
                        tunnel: w323 -> [w340]
                        tunnel: w322 -> [w339]
                        tunnel: [w338] -> w321
                        tunnel: w320 -> [w335]
                        tunnel: w319 -> [w334]
                        i -> [w337]
                        n84 = stacked-sequence {
                          seq-local: [w355 _] -> [_ w374]
                          seq-local: [w351 _] -> [_ w373]
                          tunnel: w349 -> [w364 _]
                          tunnel: w348 -> [w363 _]
                          tunnel: w347 -> [w362 _]
                          tunnel: w346 -> [w361 _]
                          tunnel: w345 -> [w359 _]
                          tunnel: [w358 _] -> w344
                          tunnel: w343 -> [_ w376]
                          tunnel: w342 -> [_ w375]
                          tunnel: w341 -> [_ _]
                          tunnel: w337 -> [w357 _]
                          tunnel: w340 -> [w353 _]
                          tunnel: w339 -> [w352 _]
                          tunnel: [_ w372] -> w338
                          tunnel: w337 -> [_ _]
                          tunnel: w336 -> [_ _]
                          tunnel: w335 -> [w350 _]
                          tunnel: w334 -> [_ w369]
                          frame #0 {
                            n85 = Equal To 0?(x=w357) -> (x = 0?=w356:bool)
                            n86 = call "zern2command_test.vi"("Initial haso file"=w361, "error in (no error)"=w352, "interaction matrix file"=w362, "Zern coef in"=w363, "Zern index in"=w364) -> ("error out"=w351:errorcluster, "Zern coef out"=w354:sgl[], "Offset positions"=w360:sgl[])  [unwired: 4 in]
                            n87 = case shown="False" w356 {
                              tunnel: [w365 w366] -> w355
                              tunnel: w354 -> [w365 _]
                              tunnel: w353 -> [_ _]
                              tunnel: w350 -> [_ w366]
                              frame False {
                              }
                              frame True {
                              }
                            }
                            n88 = Add(x=w359, y=w360) -> (x+y=w358:dbl[])
                          }
                          frame #1 {
                            n89 = Number To Fractional String(number=w369, precision (6)=0) -> (F-format string=w368:string)  [unwired: 2 in]
                            n90 = Concatenate Strings(w376, w375, "_", w368, "_coeff.txt") -> (w384:string)
                            n91 = String To Path(string=w384) -> (path=w383:path)
                            n92 = Open/Create/Replace File(file path (use dialog)=w383, error in=w373, operation (0:open)=3) -> (refnum out=w380:refnum<file>, error out=w381:errorcluster)  [unwired: 3 in, 1 out]
                            n93 = Array To Spreadsheet String(array=w374, 3:"%f") -> (spreadsheet string=w371:string)  [unwired: 1 in]
                            n94 = Set File Position(refnum=w380, from (0:start)=1, error in=w381) -> (refnum out=w378:refnum<file>, error out=w377:errorcluster)  [unwired: 1 in]
                            n95 = Write to Text File(file (use dialog)=w378, text=w371, error in=w377) -> (error out=w372:errorcluster)  [unwired: 1 in, 2 out]
                          }
                        }
                      }
                    }
                    frame #2 {
                      n96 = Number To Fractional String(number=w388, precision (6)=0) -> (F-format string=w387:string)  [unwired: 2 in]
                      n97 = Concatenate Strings(w393, w392, "_", w387, "_IniAbr+offset.txt") -> (w403:string)
                      n98 = String To Path(string=w403) -> (path=w401:path)
                      n99 = Open/Create/Replace File(file path (use dialog)=w401, error in=w391, operation (0:open)=3) -> (refnum out=w398:refnum<file>, error out=w399:errorcluster)  [unwired: 3 in, 1 out]
                      n100 = Array To Spreadsheet String(array=w394, 3:"%f") -> (spreadsheet string=w405:string)  [unwired: 1 in]
                      n101 = Set File Position(refnum=w398, from (0:start)=1, error in=w399) -> (refnum out=w396:refnum<file>, error out=w395:errorcluster)  [unwired: 1 in]
                      n102 = Write to Text File(file (use dialog)=w396, text=w405, error in=w395) -> (error out=w390:errorcluster)  [unwired: 1 in, 2 out]
                    }
                  }
                }
                frame #3 {
                  # "set andor kinetics and spooling, \nstart acquire and wait for the external trigger"
                  n103 = Number To Fractional String(number=w409, precision (6)=0) -> (F-format string=w407:string)  [unwired: 2 in]
                  n104 = Concatenate Strings(w413, w412, "_PhsDiv_ToBeDeleted_", w407) -> (w410:string)
                  n105 = call "SetSpool_WaitForExtTrigger.vi"("path and name"=w410, "Kinetic Series"=w414) -> ()  [unwired: 10 in]
                }
                frame #4 {
                  # "take phase diversity pictures"
                  n106 = for {
                    N: w421 -> [_]
                    tunnel: w426 -> [w437]
                    tunnel: w425 -> [w436]
                    tunnel: w424 -> [w435]
                    tunnel: w420 -> [w434]
                    tunnel: w423 -> [w433]
                    tunnel: w422 -> [w432] mode=indexing
                    tunnel: w419 -> [w431]
                    tunnel: w418 -> [w430]
                    tunnel: [w429] -> w416
                    tunnel: [w428] -> w417
                    tunnel: w415 -> [w427]
                    n107 = stacked-sequence {
                      seq-local: [w438 _] -> [_ w448]
                      tunnel: w437 -> [_ w445]
                      tunnel: w436 -> [_ _]
                      tunnel: w435 -> [_ _]
                      tunnel: w434 -> [_ _]
                      tunnel: w433 -> [_ _]
                      tunnel: w432 -> [w439 _]
                      tunnel: w431 -> [_ w449]
                      tunnel: w430 -> [w440 _]
                      tunnel: [_ w447] -> w429
                      tunnel: [_ w446] -> w428
                      tunnel: w427 -> [w441 _]
                      frame #0 {
                        # "response time of mirror"
                        n108 = call <userlib>:"LVClass_WavefrontCorrector Move to Absolute Position.vi"("WavefrontCorrector in"=w441, "Absolute Positions"=w439, "error in (no error)"=w440) -> ("error out"=w438:errorcluster)  [unwired: 11 in, 1 out]
                        n109 = Add(x=5, y=10) -> (x+y=w442:i32)
                        n110 = Wait (ms)(milliseconds to wait=w442) -> ()  [unwired: 1 out]
                      }
                      frame #1 {
                        n111 = for {
                          N: w445 -> [_]
                          tunnel: w449 -> [w454]
                          tunnel: w448 -> [w453]
                          tunnel: [w452] -> w447
                          tunnel: [w451] -> w446
                          tunnel: w445 -> [w450]
                          n112 = stacked-sequence {
                            tunnel: w454 -> [w459 _]
                            tunnel: w453 -> [w457 _]
                            tunnel: [w456 _] -> w452
                            tunnel: [w455 _] -> w451
                            tunnel: w450 -> [_ w464]
                            frame #0 {
                              n113 = local read "EMCCD trigger port"() -> (w462:tag)
                              n114 = Add(x=w459, y=0.04) -> (x+y=w458:dbl)
                              n115 = Multiply(x=w458, y=1000.0) -> (x*y=w455:dbl)
                              n116 = call "trig EMCCD.vi"("error in (no error)"=w457, "exp time (ms)"=w455, "lines"=w462) -> ("error out"=w456:errorcluster)
                            }
                            frame #1 {
                              n117 = Not Equal?(x=w464, y=1) -> (x != y?=w465:bool)
                              n118 = case shown="True" w465 {
                                frame False {
                                }
                                frame True {
                                n119 = Wait (ms)(milliseconds to wait=50) -> ()  [unwired: 1 out]
                                }
                              }
                            }
                          }
                        }
                      }
                    }
                  }
                }
                frame #5 {
                  # "send out a trigger to EMCCD to end the aquisition."
                  n120 = local read "EMCCD trigger port"() -> (w468:tag)
                  n121 = call "trig EMCCD.vi"("exp time (ms)"=w467, "lines"=w468) -> ()  [unwired: 1 in, 1 out]
                }
                frame #6 {
                  w476 = 0
                  w469 = 1
                  # "save phase diversity pictures:\npictures per phase*number of phases (Eg: 2*5=10 pictures in this file)"
                  n122 = Number To Fractional String(number=w479, precision (6)=w476) -> (F-format string=w475:string)  [unwired: 2 in]
                  n123 = Concatenate Strings(w480, "_", w475) -> (w471:string)
                  n124 = Concatenate Strings(w471, ".tif") -> (w472:string)
                  n125 = Concatenate Strings(w478, w472) -> (w474:string)
                  n126 = call <userlib>:"SaveAsTiffEx.vi"("path"=w474, "palette"="C:\\Program Files\\Andor SOLIS\\GREY.PAL", "position"=w476, "type"=w469, "mode"=w469) -> ()  [unwired: 13 in, 2 out]
                }
                frame #7 {
                  # "offset+ini path and name no.tif"
                  # "groundtruth path and name no.tif"
                  # "take a picture of groundtruth and offset+ini abbr, and cal imq for each"
                  n127 = stacked-sequence {
                    seq-local: [w492 _ _ _] -> [_ w505 _ _]
                    seq-local: [_ _ w508 _] -> [_ _ _ w521]
                    tunnel: w490 -> [w497 _ w514 _]
                    tunnel: w489 -> [w496 _ w513 _]
                    tunnel: w488 -> [w495 _ w512 _]
                    tunnel: w487 -> [w494 _ w511 _]
                    tunnel: w484 -> [_ _ w510 _]
                    tunnel: w486 -> [w493 _ w509 _]
                    tunnel: w485 -> [_ w506 _ w524]
                    tunnel: [_ w502 _ _] -> w483
                    tunnel: w482 -> [w491 _ _ _]
                    tunnel: [_ _ _ w519] -> w481
                    frame #0 {
                      # "take a picture of groundtruth"
                      n128 = Number To Fractional String(number=w495, precision (6)=0) -> (F-format string=w498:string)  [unwired: 2 in]
                      n129 = Concatenate Strings(w497, w496, "_grdtrth_", w498) -> (w492:string)
                      n130 = call "Apply DM command and take picture.vi"("WavefrontCorrector in"=w493, "Offset positions"=w491, "trigger time (ms)"=w494, "# of pictures"=1, "path and file name, no .tif at the end"=w492) -> ()  [unwired: 6 in, 1 out]
                    }
                    frame #1 {
                      # "calculate imq of groundtruth"
                      n131 = Concatenate Strings(w505, ".tif") -> (w503:string)
                      n132 = call "MATLAB image quality metrics.vi"("Background Value"=w506, "File Path and Name w/.tif"=w503, "Metrics Type"="Metrics Type") -> ("image quality"=w502:dbl)  [unwired: 8 in]
                      "groundtruth image quality value" <- w502
                    }
                    frame #2 {
                      # "take a picture of offset+ini abbr"
                      n133 = Number To Fractional String(number=w512, precision (6)=0) -> (F-format string=w515:string)  [unwired: 2 in]
                      n134 = Concatenate Strings(w514, w513, "_abbr_", w515) -> (w508:string)
                      n135 = call "Apply DM command and take picture.vi"("WavefrontCorrector in"=w509, "Offset positions"=w510, "trigger time (ms)"=w511, "# of pictures"=1, "path and file name, no .tif at the end"=w508) -> ()  [unwired: 6 in, 1 out]
                    }
                    frame #3 {
                      # "calculate imq of offset+ini"
                      n136 = local read "Metrics Type"() -> (w520:T3)
                      n137 = Concatenate Strings(w521, ".tif") -> (w522:string)
                      n138 = call "MATLAB image quality metrics.vi"("Background Value"=w524, "File Path and Name w/.tif"=w522, "Metrics Type"=w520) -> ("image quality"=w519:dbl)  [unwired: 8 in]
                      "aberrated image quality value" <- w519
                    }
                  }
                }
                frame #8 {
                  # "run matlab correction?"
                  n139 = case shown="True" w539 {
                    tunnel: w544 -> [_ w569]
                    tunnel: w545 -> [_ w568]
                    tunnel: w543 -> [_ w567]
                    tunnel: w542 -> [_ w566]
                    tunnel: w529 -> [_ w565]
                    tunnel: w541 -> [_ w564]
                    tunnel: w540 -> [_ w563]
                    tunnel: w528 -> [_ w562]
                    tunnel: w538 -> [_ _]
                    tunnel: [0 w561] -> w537
                    tunnel: w536 -> [_ w560]
                    tunnel: [errorcluster {"status"=FALSE, "code"=0, "source"=""} ("Error out 2") w559] -> w535
                    tunnel: w534 -> [_ w558]
                    tunnel: w533 -> [_ w557]
                    tunnel: w532 -> [_ _]
                    tunnel: w531 -> [_ w556]
                    tunnel: w530 -> [_ w553]
                    tunnel: w529 -> [_ w555]
                    tunnel: w528 -> [_ w554]
                    tunnel: w527 -> [_ w551]
                    tunnel: w526 -> [_ w550]
                    tunnel: [dbl[] [] w549] -> w525
                    frame False {
                    }
                    frame True {
                      # "matlab reconstructed Zern"
                      n140 = stacked-sequence {
                        seq-local: [w583 _ _ _ _ _ _ _ _ _ _] -> [_ _ _ _ _ _ w726 _ _ _ _]
                        seq-local: [w585 _ _ _ _ _ _ _ _ _ _] -> [_ _ _ _ _ _ w722 _ _ _ _]
                        seq-local: [_ _ _ _ w705 _ _ _ _ _ _] -> [_ _ _ _ _ w712 _ _ _ _ _]
                        seq-local: [_ _ w693 _ _ _ _ _ _ _ _] -> [_ _ _ w700 _ _ _ _ _ _ _]
                        seq-local: [_ _ _ w702 _ _ _ _ _ _ _] -> [_ _ _ _ w706 _ _ _ _ _ _]
                        seq-local: [_ w685 _ _ _ _ _ _ _ _ _] -> [_ _ _ _ _ _ _ _ _ _ w760]
                        tunnel: w569 -> [w584 w688 _ _ _ _ _ _ _ w750 _]
                        tunnel: w568 -> [w582 w687 _ _ _ _ _ _ _ w749 _]
                        tunnel: w567 -> [w574 _ _ _ _ _ w725 _ _ _ _]
                        tunnel: w566 -> [w577 _ _ _ w707 _ w724 _ _ _ _]
                        tunnel: w565 -> [_ _ _ w704 _ w714 _ w732 w746 _ _]
                        tunnel: w563 -> [_ _ w694 _ _ _ _ _ _ _ _]
                        tunnel: [_ _ _ w703 _ _ _ _ _ _ _] -> _
                        tunnel: w564 -> [_ _ _ w703 _ _ _ w731 _ _ _]
                        tunnel: w562 -> [w581 w686 _ _ _ _ _ _ _ w751 _]
                        tunnel: [w580 _ _ _ _ _ _ _ _ _ _] -> w561
                        tunnel: w560 -> [_ _ w695 _ _ _ _ _ _ _ _]
                        tunnel: [_ _ _ _ _ _ _ w730 _ _ _] -> w559
                        tunnel: w558 -> [w571 _ w696 _ w708 _ w718 _ _ _ _]
                        tunnel: w557 -> [_ w689 _ _ _ _ _ _ _ _ w758]
                        tunnel: w556 -> [w579 _ _ _ _ _ _ _ _ _ _]
                        tunnel: w555 -> [w576 _ _ _ _ _ _ _ _ _ _]
                        tunnel: w554 -> [w575 _ _ _ _ _ _ _ _ _ _]
                        tunnel: 2 -> [w578 _ _ _ _ _ _ _ _ _ _]
                        tunnel: w553 -> [w573 _ _ _ _ _ _ _ _ _ _]
                        tunnel: w551 -> [w572 _ _ _ _ _ _ _ _ _ _]
                        tunnel: w550 -> [_ _ _ _ _ _ w715 _ _ _ _]
                        tunnel: [w570 _ _ _ _ _ _ _ _ _ _] -> w549
                        frame #0 {
                          n141 = while {
                            tunnel: [w605] -> w585
                            tunnel: w584 -> [w604]
                            tunnel: [w603] -> w583
                            tunnel: w582 -> [w602]
                            tunnel: w581 -> [w601]
                            tunnel: [w600] -> w580
                            tunnel: w579 -> [w599]
                            shift-right: [w590] -> _
                            shift-left: w578 -> [w598]
                            tunnel: w577 -> [w597]
                            tunnel: w576 -> [w596]
                            tunnel: w575 -> [w595]
                            tunnel: w574 -> [w594]
                            tunnel: w573 -> [w593]
                            tunnel: w572 -> [w588]
                            tunnel: w571 -> [w587]
                            tunnel: [w586] -> w570 mode=indexing
                            stop <- w591 stop-if-true
                            n142 = stacked-sequence {
                              seq-local: [w614 _ _ _] -> [_ w648 _ _]
                              seq-local: [_ w650 _ _] -> [_ _ w666 _]
                              seq-local: [w613 _ _ _] -> [_ w647 _ _]
                              tunnel: [w613 _ _ _] -> w605
                              tunnel: w604 -> [w633 w651 _ _]
                              tunnel: [w614 _ _ _] -> w603
                              tunnel: w602 -> [w610 w649 _ _]
                              tunnel: w601 -> [w627 _ _ _]
                              tunnel: [w617 _ _ _] -> w600
                              tunnel: w599 -> [w615 _ w667 _]
                              tunnel: w598 -> [w612 w643 _ w679]
                              tunnel: w597 -> [_ w646 _ _]
                              tunnel: w596 -> [_ w645 _ _]
                              tunnel: w595 -> [_ w644 _ _]
                              tunnel: w594 -> [_ w642 _ _]
                              tunnel: w593 -> [_ _ w665 _]
                              tunnel: [_ _ w664 _] -> w592
                              tunnel: [_ _ _ w674] -> w590
                              tunnel: [_ _ _ w671] -> w589
                              tunnel: w588 -> [_ w641 _ _]
                              tunnel: w587 -> [_ w640 _ _]
                              tunnel: [_ _ w663 _] -> w586
                              frame #0 {
                                w607 = "_"
                                # "MATLAB does the reconstruction, written by Min Guo"
                                # "other parameters are default in this VI"
                                n143 = Number To Fractional String(number=w627, precision (6)=0) -> (F-format string=w606:string)  [unwired: 2 in]
                                n144 = Concatenate Strings(w610, "_", w606) -> (w616:string)
                                n145 = String To Path(string=w633) -> (path=w634:path)
                                n146 = Number To Fractional String(number=w612, precision (6)=0) -> (F-format string=w609:string)  [unwired: 2 in]
                                n147 = Concatenate Strings(w633, w610, w607, w609, "ImgCorr", w607, w606) -> (w632:string)
                                n148 = String To Path(string=w632) -> (path=w631:path)
                                n149 = call "recon_zern_fileIO_MATLAB_v2.vi"("Number of Phase"=w612, "Number for average"="Number for average", "Crop Size of image"="Crop Size of image", "Background Value"=w615, "Zernike Order"="Zernike Order", "Use GPU"="Use GPU", "Iteration Number"="Iteration Number", "File Name"=w616, "Gamma Value"="Gamma Value", "Path In"=w634, "Show Input"="Show Input", "Path Out"=w631, "Show Recon"="Show Recon") -> ("Zern coef out"=w629:sgl[], "RMSE Value"=w617:dbl, "error out"=w613:errorcluster)  [unwired: 3 in, 1 out]
                                n150 = case shown="True" "Keep Reconstructed Defocus component?" {
                                tunnel: w629 -> [w635 w639]
                                tunnel: [w635 w636] -> w614
                                frame False {
                                }
                                frame True {
                                n151 = Replace Array Subset(array=w639, new element=0.0, index=2) -> (w636:sgl[])
                                }
                                }
                              }
                              frame #1 {
                                w653 = 0
                                w662 = 1
                                # "? sign\n? indicator corrcoeff+offsetiniabbr"
                                # "get correction command\ntake a picture"
                                n152 = call-poly <vilib>:"Ramp Pattern.vi"("start"=w662, "end"=32, "delta"=w662) -> ("Ramp Pattern"=w660:dbl[])  [unwired: 6 in, 2 out]
                                n153 = call "zern2command_test.vi"("Initial haso file"=w641, "error in (no error)"=w647, "interaction matrix file"=w642, "Zern coef in"=w648, "Zern index in"=w660) -> ("Offset positions"=w659:sgl[])  [unwired: 4 in, 2 out]
                                n154 = Add(x=w646, y=w659) -> (x+y=w658:dbl[])
                                n155 = Number To Fractional String(number=w644, precision (6)=w653) -> (F-format string=w655:string)  [unwired: 2 in]
                                n156 = Number To Fractional String(number=w643, precision (6)=w653) -> (F-format string=w652:string)  [unwired: 2 in]
                                n157 = Concatenate Strings(w651, w649, "_", w652, "ImgCorr_", w655) -> (w650:string)
                                n158 = call "Apply DM command and take picture.vi"("WavefrontCorrector in"=w640, "Offset positions"=w658, "trigger time (ms)"=w645, "# of pictures"=1, "path and file name, no .tif at the end"=w650) -> ()  [unwired: 6 in, 1 out]
                              }
                              frame #2 {
                                n159 = local read "Metrics Type"() -> (w668:T3)
                                n160 = Concatenate Strings(w666, ".tif") -> (w669:string)
                                n161 = call "MATLAB image quality metrics.vi"("Background Value"=w667, "File Path and Name w/.tif"=w669, "Metrics Type"=w668) -> ("image quality"=w663:dbl)  [unwired: 8 in]
                                n162 = Greater?(x=w663, y=w665) -> (0:w664:bool)
                              }
                              frame #3 {
                                n163 = Equal?(x="number of phase div image", y=0.9) -> (x = y?=w675:bool)
                                n164 = To Byte Integer(number="number of phase div image") -> (8bit integer=w678:i8)
                                n165 = Add(x=w679, y=w678) -> (x+y=w674:i32)
                                n166 = case shown="False" w675 {
                                tunnel: w674 -> [_ w683]
                                tunnel: [FALSE w682] -> w672
                                frame False {
                                }
                                frame True {
                                n167 = Greater?(x=w683, y=3) -> (0:w682:bool)
                                }
                                }
                                n168 = Greater?(x=w674, y=5) -> (0:w673:bool)
                                n169 = Or(x=w673, y=w672) -> (x .or. y?=w671:bool)
                              }
                            }
                            n170 = Or(x=w592, y=w589) -> (x .or. y?=w591:bool)
                          }
                        }
                        frame #1 {
                          # "set andor kinetics and spooling, \nstart acquire and wait for the external trigger"
                          n171 = Number To Fractional String(number=w686, precision (6)=0) -> (F-format string=w690:string)  [unwired: 2 in]
                          n172 = Concatenate Strings(w688, w687, "_Corr_ToBeDeleted_", w690) -> (w685:string)
                          n173 = call "SetSpool_WaitForExtTrigger.vi"("path and name"=w685, "Kinetic Series"=w689) -> ()  [unwired: 10 in]
                        }
                        frame #2 {
                          # "groundtruth command"
                          # "response time of mirror"
                          n174 = call <userlib>:"LVClass_WavefrontCorrector Move to Absolute Position.vi"("WavefrontCorrector in"=w696, "Absolute Positions"=w695, "error in (no error)"=w694) -> ("error out"=w693:errorcluster)  [unwired: 11 in, 1 out]
                          n175 = Add(x=5, y=10) -> (x+y=w697:i32)
                          n176 = Wait (ms)(milliseconds to wait=w697) -> ()  [unwired: 1 out]
                        }
                        frame #3 {
                          # "take offset/groundtruth picture, only one"
                          n177 = local read "EMCCD trigger port"() -> (w701:tag)
                          n178 = call "trig EMCCD.vi"("error in (no error)"=w700, "exp time (ms)"=w704, "lines"=w701) -> ("error out"=w702:errorcluster)
                        }
                        frame #4 {
                          # "aberrated picture command"
                          # "response time of mirror"
                          n179 = call <userlib>:"LVClass_WavefrontCorrector Move to Absolute Position.vi"("WavefrontCorrector in"=w708, "Absolute Positions"=w707, "error in (no error)"=w706) -> ("error out"=w705:errorcluster)  [unwired: 11 in, 1 out]
                          n180 = Add(x=5, y=10) -> (x+y=w709:i32)
                          n181 = Wait (ms)(milliseconds to wait=w709) -> ()  [unwired: 1 out]
                        }
                        frame #5 {
                          # "take offset+initial aberr picture, only one"
                          n182 = local read "EMCCD trigger port"() -> (w713:tag)
                          n183 = call "trig EMCCD.vi"("error in (no error)"=w712, "exp time (ms)"=w714, "lines"=w713) -> ()  [unwired: 1 out]
                        }
                        frame #6 {
                          w729 = 1
                          # "correction command"
                          # "response time of mirror"
                          n184 = call-poly <vilib>:"Ramp Pattern.vi"("start"=w729, "end"=32, "delta"=w729) -> ("Ramp Pattern"=w727:dbl[])  [unwired: 6 in, 2 out]
                          n185 = call "zern2command_test.vi"("Initial haso file"=w715, "error in (no error)"=w722, "interaction matrix file"=w725, "Zern coef in"=w726, "Zern index in"=w727) -> ("error out"=w716:errorcluster, "Offset positions"=w723:sgl[])  [unwired: 4 in, 1 out]
                          n186 = Add(x=w724, y=w723) -> (x+y=w717:dbl[])
                          n187 = call <userlib>:"LVClass_WavefrontCorrector Move to Absolute Position.vi"("WavefrontCorrector in"=w718, "Absolute Positions"=w717, "error in (no error)"=w716) -> ()  [unwired: 11 in, 2 out]
                          n188 = Add(x=5, y=10) -> (x+y=w719:i32)
                          n189 = Wait (ms)(milliseconds to wait=w719) -> ()  [unwired: 1 out]
                        }
                        frame #7 {
                          # "corrected pictures"
                          n190 = for {
                            N: w731 -> [w733]
                            tunnel: w732 -> [w736]
                            shift-right: [w734] -> w730
                            shift-left: _ -> [w735]
                            n191 = stacked-sequence {
                              tunnel: w736 -> [w739 _]
                              tunnel: w735 -> [w738 _]
                              tunnel: [w737 _] -> w734
                              tunnel: w733 -> [_ w741]
                              frame #0 {
                                n192 = local read "EMCCD trigger port"() -> (w740:tag)
                                n193 = call "trig EMCCD.vi"("error in (no error)"=w738, "exp time (ms)"=w739, "lines"=w740) -> ("error out"=w737:errorcluster)
                              }
                              frame #1 {
                                n194 = Not Equal?(x=w741, y=1) -> (x != y?=w743:bool)
                                n195 = case shown="True" w743 {
                                frame False {
                                }
                                frame True {
                                n196 = Wait (ms)(milliseconds to wait=50) -> ()  [unwired: 1 out]
                                }
                                }
                              }
                            }
                          }
                        }
                        frame #8 {
                          # "one more trigger to end picture acquisition"
                          n197 = local read "EMCCD trigger port"() -> (w745:tag)
                          n198 = call "trig EMCCD.vi"("exp time (ms)"=w746, "lines"=w745) -> ()  [unwired: 1 in, 1 out]
                        }
                        frame #9 {
                          w754 = 0
                          w747 = 1
                          # "save:\none groundtruth picture\none offset+abrr picture\nPictures per phase*corrected picture"
                          n199 = Number To Fractional String(number=w751, precision (6)=w754) -> (F-format string=w753:string)  [unwired: 2 in]
                          n200 = Concatenate Strings(w749, "_grdtrth_abrr_Corr_", w753, ".tif") -> (w757:string)
                          n201 = Concatenate Strings(w750, w757) -> (w752:string)
                          n202 = call <userlib>:"SaveAsTiffEx.vi"("path"=w752, "palette"="C:\\Program Files\\Andor SOLIS\\GREY.PAL", "position"=w754, "type"=w747, "mode"=w747) -> ()  [unwired: 13 in, 2 out]
                        }
                        frame #10 {
                          n203 = case shown="True" TRUE {
                            tunnel: w760 -> [_ w762]
                            tunnel: w758 -> [_ w761]
                            frame False {
                            }
                            frame True {
                              # "delete spooling data"
                              n204 = for {
                                N: w761 -> [_]
                                tunnel: w762 -> [w769]
                                i -> [w767]
                                n205 = Number To Fractional String(number=w767, precision (6)=0) -> (F-format string=w765:string)  [unwired: 2 in]
                                n206 = Concatenate Strings(w769, "000000000", w765, ".dat") -> (w764:string)
                                n207 = String To Path(string=w764) -> (path=w770:path)
                                n208 = Delete(path (use dialog)=w770) -> ()  [unwired: 4 in, 3 out]
                              }
                            }
                          }
                        }
                      }
                      "Corrected Image Quality Value" <- w549
                    }
                  }
                }
                frame #9 {
                  # "delete spooling data of phase diversity"
                  n209 = case shown="True" TRUE {
                    tunnel: w773 -> [_ w775]
                    tunnel: w771 -> [_ w774]
                    frame False {
                    }
                    frame True {
                      n210 = for {
                        N: w774 -> [_]
                        tunnel: w775 -> [w781]
                        i -> [w779]
                        n211 = Greater?(x=w779, y=9) -> (0:w777:bool)
                        n212 = Number To Fractional String(number=w779, precision (6)=0) -> (F-format string=w783:string)  [unwired: 2 in]
                        n213 = case shown="False" w777 {
                          tunnel: ["000000000" "00000000"] -> w776
                          frame False {
                          }
                          frame True {
                          }
                        }
                        n214 = Concatenate Strings(w781, w776, w783, ".dat") -> (w780:string)
                        n215 = String To Path(string=w780) -> (path=w785:path)
                        n216 = Delete(path (use dialog)=w785) -> ()  [unwired: 4 in, 3 out]
                      }
                    }
                  }
                }
                frame #10 {
                  w802 = "\r"
                  # "save image quality values"
                  n217 = local read "number of phase div image"() -> (w796:dbl)
                  n218 = local read "Metrics Type"() -> (w814:T3)
                  n219 = case shown="\" \", Default" w814 {
                    tunnel: [" \" \", Default." " \"max intensity\"." " \"mean intensity\"." " \"RMS contrast\"." " \"sharpness - image domain\"." " \"sharpness - spectral domain 1: 0~r0\"." " \"sharpness - spectral domain 2: 0.1*r0~0.5*r0\"." " \"norm DCT  - spectral domain 3: 0~r0\"."] -> w812
                    frame " ", Default {
                    }
                    frame "max intensity" {
                    }
                    frame "mean intensity" {
                    }
                    frame "RMS contrast" {
                    }
                    frame "sharpness - image domain" {
                    }
                    frame "sharpness - spectral domain 1: 0~r0" {
                    }
                    frame "sharpness - spectral domain 2: 0.1*r0~0.5*r0" {
                    }
                    frame "norm DCT  - spectral domain 3: 0~r0" {
                    }
                  }
                  n220 = Multiply(x=w796, y=10.0) -> (x*y=w788:dbl)
                  n221 = case shown="20" w788 {
                    tunnel: ["" "2-, 3-, 4- and 5-phase-corrected." "2- and 3-phase-corrected." "2- and 4-phase-corrected." "2- and 5-phase-corrected."] -> w795
                    frame 0, Default {
                    }
                    frame 10 {
                    }
                    frame 9 {
                    }
                    frame 20 {
                    }
                    frame 29 {
                    }
                  }
                  n222 = Concatenate Strings(w792, w791, "_ImageQuality.txt") -> (w789:string)
                  n223 = String To Path(string=w789) -> (path=w794:path)
                  n224 = Number To Fractional String(number=w808, precision (6)=8) -> (F-format string=w806:string)  [unwired: 2 in]
                  n225 = Number To Fractional String(number=w800, precision (6)=8) -> (F-format string=w799:string[])  [unwired: 2 in]
                  n226 = Number To Fractional String(number=w804, precision (6)=8) -> (F-format string=w803:string)  [unwired: 2 in]
                  n227 = Concatenate Strings("This data set uses metrics:  ", w812, w802, "The image quality value of groundtruth is ", w806, w802, "The image quality value of offset+manual abberation is ", w803, w802, "The image quality value of corrected is ", w799, " for ", w795) -> (w793:string)
                  n228 = Write to Text File(file (use dialog)=w794, text=w793) -> ()  [unwired: 2 in, 3 out]
                }
              }
            }
          }
          frame #2 {
            # "shut down shutter of 488nm laser"
            n229 = invoke class="MG17Motor" method="SC_Disable"(reference=w831, "lChanID"=w830) -> (reference out=w829:refnum<k7>, "lChanID"=w828:i32)  [unwired: 2 in, 2 out]
          }
          frame #3 {
            # "save the RMS of (calculated zer-real zer)"
            n230 = Concatenate Strings(w834, w833, "_RMSE.txt") -> (w839:string)
            n231 = String To Path(string=w839) -> (path=w838:path)
            n232 = Number To Fractional String(number=w835) -> (F-format string=w836:string[])  [unwired: 3 in]
            n233 = Write to Text File(file (use dialog)=w838, text=w836) -> (error out=w832:errorcluster)  [unwired: 2 in, 2 out]
          }
        }
        n234 = Merge Errors(w201, w200, w195) -> (w194:errorcluster)
        "Error out" <- w194
        n235 = Unbundle(w194) -> ("status"=w190:bool)  [unwired: 2 out]
        n236 = case shown="True" w190 {
          tunnel: [w216 w217] -> w193
          tunnel: w190 -> [w215 w217]
          frame False {
            n237 = Not(x=w215) -> (.not. x?=w216:bool)
          }
          frame True {
          }
        }
        n238 = Or(x=w193, y="?") -> (x .or. y?=w191:bool)
      }
    }
    frame #4 {
      n239 = case shown="True" "Turn off EMCCD when finished?" {
        frame False {
        }
        frame True {
          n240 = flat-sequence {
            frame #0 {
              n241 = call <userlib>:"CoolerOFF.vi"() -> ()  [unwired: 2 in, 2 out]
            }
            frame #1 {
              # "shut down EMCCD"
              n242 = call <userlib>:"ShutDown.vi"() -> ()  [unwired: 2 in, 2 out]
            }
          }
        }
      }
    }
    frame #5 {
      # "if not \"stop control\", the shutter can be control when the program is not running"
      # "shut down casao"
      n243 = call <userlib>:"LVClass_WavefrontCorrector dtor.vi"("WavefrontCorrector in"=w845, "error in (no error)"=w843) -> ("error out"=w842:errorcluster)  [unwired: 12 in, 1 out]
      n244 = call <userlib>:"LVClass_WavefrontCorrectorSet dtor.vi"("WavefrontCorrectorSet in"=w844, "error in (no error)"=w842) -> ()  [unwired: 12 in, 2 out]
      n245 = case shown="True" FALSE {
        tunnel: w846 -> [_ w847]
        frame False {
        }
        frame True {
          n246 = invoke class="MG17Motor" method="StopCtrl"(reference=w847) -> ()  [unwired: 2 in, 3 out]
        }
      }
    }
  }
